vi "PH_Sequencer.ProcCases.vi"(0 "i ref in":refnum<vi>, 1 "selector":string, 2 "Data":T1, 3 "call cluster":T2={"Object"="", "Selector"="", "CallType"=enum."synchronous", "Async Object"="", "Async Selector"="", "Data Descriptor"="", "Data"=[], "Error #"=0, "Expire"=0}, 5 "error in (no error)":errorcluster) -> (14 "i ref out":refnum<vi>, 17 "answer cluster":T2={"Object"="", "Selector"="", "CallType"=enum."synchronous", "Async Object"="", "Async Selector"="", "Data Descriptor"="", "Data"=[], "Error #"=0, "Expire"=0}, 19 "error out":errorcluster)   [LabVIEW 2014, in "PH_Sequencer.lvlib"]
doc: "This method is called by a process from within the default case in the event loop. The methods of a class that are linked to events will be called from THIS method. Add your code here."
uses:
  PH_Sequencer.lvlib
  CSCore/CSSystem/CoreDefs/CoreDefs.call_type.ctl
  CSCore/BaseProcess/BaseProcess.descriptor string definition.ctl
  CSCore/CSSystem/CoreDefs/CoreDefs.rawDataType.ctl
  PH_Timing/PH_Timing.Slow Trigger Settings.ctl
  PH_Timing/PH_Timing.Phase FEs.ctl
  PH_Timing/PH_Timing.Timing Mode.ctl
  CSCore/CSSystem/CSSystemLib/CSSystemLib.object condition.ctl
  CSCore/CSSystem/CoreLib/CoreLib.string 2 byte array.vi
  CSCore/CSSystem/CoreLib/CoreLib.byte array 2 double.vi
  CSCore/CSSystem/CoreLib/CoreLib.byte array 2 short.vi
  CSCore/CSSystem/CoreLib/CoreLib.byte array 2 string.vi
  CSCore/BaseProcess/BaseProcess.lvlib
  CSCore/CAEObj/CAEObj.lvlib
  CSCore/CSSystem/CoreLib/CoreLib.lvlib
  CSCore/CSSystem/CSSystemLib/CSSystemLib.lvlib
  PH_Timing/PH_Timing.lvlib
  PH_Common/PH_Common.lvlib
  PH_PSDBController/PH_PSDBController.lvlib
  PH_PowerUnit_BaseClass/PH_PowerUnit_BaseClass.lvlib
  lib.lib/DimLVEvent/LVDimInterface/LVDimInterface.lvlib
  PH_StatusHandler/PH_StatusHandler.lvlib
  PH_PSDBWriter/PH_PSDBWriter.lvlib
  PH_SystemInformation/PH_SystemInformation.lvlib
  PH_BL-Master/PH_BL-Master.lvlib
  PH_4_Pos_Selector/PH_4_Pos_Selector.lvlib
  PH_BeamlineInformation/PH_BeamlineInformation.lvlib
  PH_BeamlineController/PH_BeamlineController.lvlib
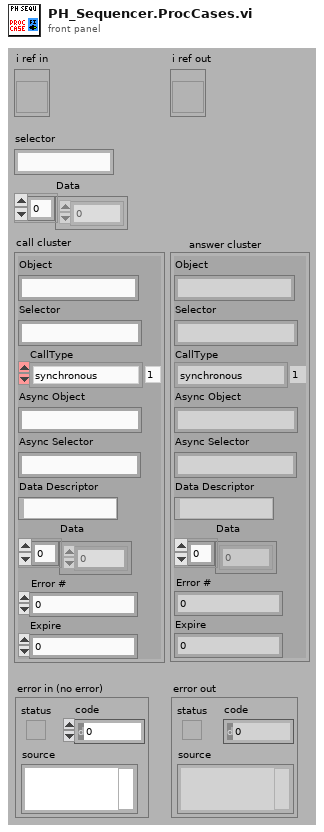
[diagram p1: front panel]
types:
  T1 = typedef "CoreDefs.rawDataType.ctl" = i8[]
  T2 = typedef "CoreDefs.call_type.ctl" = cluster{"Object":string, "Selector":string, "CallType":enum16{"simple", "synchronous", "asynchronous"}, "Async Object":string, "Async Selector":string, "Data Descriptor":T3, "Data":T1, "Error #":i32, "Expire":u32}
  T3 = typedef "BaseProcess.lvlib/BaseProcess.descriptor string definition.ctl" = string
  T4 = typedef "PH_Timing.lvlib/PH_Timing.Slow Trigger Settings.ctl" = cluster{"Delay":dbl, "externally triggered?":bool}
  T5 = typedef "PH_Timing.lvlib/PH_Timing.Phase FEs.ctl" = cluster{"Phase":dbl}
  T6 = typedef "PH_Timing.lvlib/PH_Timing.Timing Mode.ctl" = cluster{"T2":i16, "Modeselector":enum32{"10 Hz", "0.5 Hz", "Shot"}}
  T7 = typedef "PH_Sequencer.lvlib/PH_Sequencer.i attribute.ctl" = cluster{"GUI Refs":cluster{"Main Off":refnum<vi>, "Fire":refnum<vi>, "Status":refnum<vi>, "Ready":refnum<vi>, "Waiting Time":refnum<vi>, "Timeout":refnum<vi>, "PPMA Ready":refnum<vi>, "Sequencer SM State":refnum<vi>, "PPPA Ready":refnum<vi>, "Calorimeter":refnum<vi>, "Beamline Ready":refnum<vi>, "Clear Beamline":refnum<vi>, "Linkage PPMA Rods":refnum<vi>, "Linkage Current PA":refnum<vi>, "Linkage Current MA":refnum<vi>, "Timing Ready":refnum<vi>, "State Timing":refnum<vi>, "Force Timing":refnum<vi>, "PSDB Shot Comment":refnum<vi>, "State PA Backreflection":refnum<vi>, "Beamline Z6 Ready":refnum<vi>, "Clear Z6 Beamline":refnum<vi>, "Sequence length":refnum<vi>, "Timing Mode":refnum<vi>, "Slow Trigger Settings":refnum<vi>, "Experiment Description":refnum<vi>, "State PSDB":refnum<vi>, "PSDB Ready":refnum<vi>, "Set PSDB Settings":refnum<vi>, "Get PSDB Info":refnum<vi>, "Take Snapshot":refnum<vi>, "Shottype":refnum<vi>, "Experiment":refnum<vi>, "Phase Frontends":refnum<vi>, "PP 45mm PILC in use":refnum<vi>}, "Status Info":cluster{"Machine Status":T8, "WaitingTime":i32, "Timeout":bool}, "Readyness":cluster{"Ready to shot":bool, "PPMA Ready":bool, "PPPA Ready":bool, "BL Ready":bool, "Timing Ready":bool, "BL Z6 Ready":bool, "PSDBReady":bool}, "Instancenames":cluster{"PPMA Rods":string, "PP Current Meas":string, "PH Beamline Chief":string, "PA Backrefl Meas":string, "Z6 Beamline Chief":string}, "Data to read":bool, "Calorimeter":cluster{"Instancename":string, "On":bool, "linked":bool}, "Linkage":cluster{"PPMA Rods":bool, "PP Current Meas":bool, "PHELIX Beamline Chief":bool, "PA Backrefl Meas":bool, "Z6 Beamline Chief":bool}, "Timing":cluster{"Instance":string, "linked":bool, "Status":T8, "Timing Mode":T6, "Slow Trigger Settings":T4, "Info available":cluster{"ext SlowTrigger":bool, "T2":bool, "Mode":bool, "Delay Slow Trigger":bool, "Phase FEs":bool}, "FE Phase":T5}, "Service ID R2S":i32, "PSDB":cluster{"Controller Instance":string, "Controller Status":T8, "Controller linked":bool, "Settings acknowledged":bool, "Current Experiment ID":i16, "Current Shot Type":i16, "Current Comment":string, "Remember Settings":bool, "Write 2 early":bool}, "PSDB Data":cluster{"Main Off?":bool, "Sequence Length":dbl, "Sequence startet":timestamp}, "6P 4Q Positions":cluster{"Instancename":string, "linked":bool, "Position":T9}[], "PUs":T10[]}
  T8 = typedef "PH_StatusHandler.lvlib/PH_StatusHandler.Status.ctl" = i16
  T9 = typedef "PH_4_Pos_Selector.lvlib/PH_4_Pos_Selector.Position Selector.ctl" = u16
  T10 = typedef "PH_Sequencer.lvlib/PH_Sequencer.Head.ctl" = cluster{"PowerUnit":T11, "GUI Ref":refnum<vi>, "Information":T12, "linked?":bool, "GUI Ref Current Voltage":refnum<vi>}
  T11 = typedef "PH_PP_Common.lvlib/PH_PP_Common.PUs.ctl" = enum16{"no Info", "PA-19mm-1", "PA-19mm-2", "PA-45mm-PILC", "PA-45mm-MAIN", "MA-PU-1", "MA-PU-2", "MA-PU-3", "MA-PU-4", "MA-PU-5", "MA-PU-6", "MA-FR", "MA-PILC", "PA-45mm-DP"}
  T12 = typedef "PH_Sequencer.lvlib/PH_Sequencer.PU Information.ctl" = cluster{"State":T8, "Waiting Time [s]":dbl, "PU State SM":T13, "PU Timeout SM":T13}
  T13 = typedef "PH_PowerUnit_BaseClass.lvlib/PH_PowerUnit_BaseClass.SM States.ctl" = enum16{".", "Stand by", "Switch PU on", "Configure", "Set Default Voltage", "Set STANDBY", "Set READY", "Wait for Shot Cmd", "Open Dump Rods", "Open Ross Relais", "Close Ross Relais", "Switch PSU on", "Switch PSU off", "Charge", "Switch GD Channel on", "Close Dump Rods", "Rods-TO", "RR-TO", "PSU-TO", "Trigger-TO"}
  T14 = typedef "PH_SystemInformation.lvlib/PH_SystemInformation.i attribute.ctl" = cluster{"Laser Enabling":cluster{"GUI Ref":refnum<vi>, "Enabling State":T15}, "PreAmp Enabling":cluster{"GUI Ref":refnum<vi>, "Enabling State":T15}, "MainAmp Enabling":cluster{"GUI Ref":refnum<vi>, "Enabling State":T15}, "Emergency Off":cluster{"GUI Ref":refnum<vi>, "State":enum16{"no info", "off/false", "Alarm"}}, "Enabling Exp. 1":cluster{"GUI Ref":refnum<vi>, "Enabling State":T15}, "Enabling Exp. 2":cluster{"GUI Ref":refnum<vi>, "Enabling State":T15}, "Enabling Exp. 3":cluster{"GUI Ref":refnum<vi>, "Enabling State":T15}, "Enabling Exp. 4":cluster{"GUI Ref":refnum<vi>, "Enabling State":T15}, "Timing Mode":cluster{"GUI Ref":refnum<vi>, "PHELIX_Timing_Mode":enum32{"10 Hz", "0.5 Hz", "Shot"}}}
  T15 = typedef "PH_SystemInformation.lvlib/PH_SystemInformationEnabling State.ctl" = i32
  T16 = typedef "CSSystemLib.lvlib/CSSystemLib.object condition.ctl" = i32
  T17 = typedef "PH_PSDBWriter.lvlib/PH_PSDBWriter.PHELIX-Subsystems.ctl" = i32
  T18 = enum16{"Laser", "PreAmp", "MainAmp", "Exp 1", "Exp 2", "Exp 3", "Exp 4"}
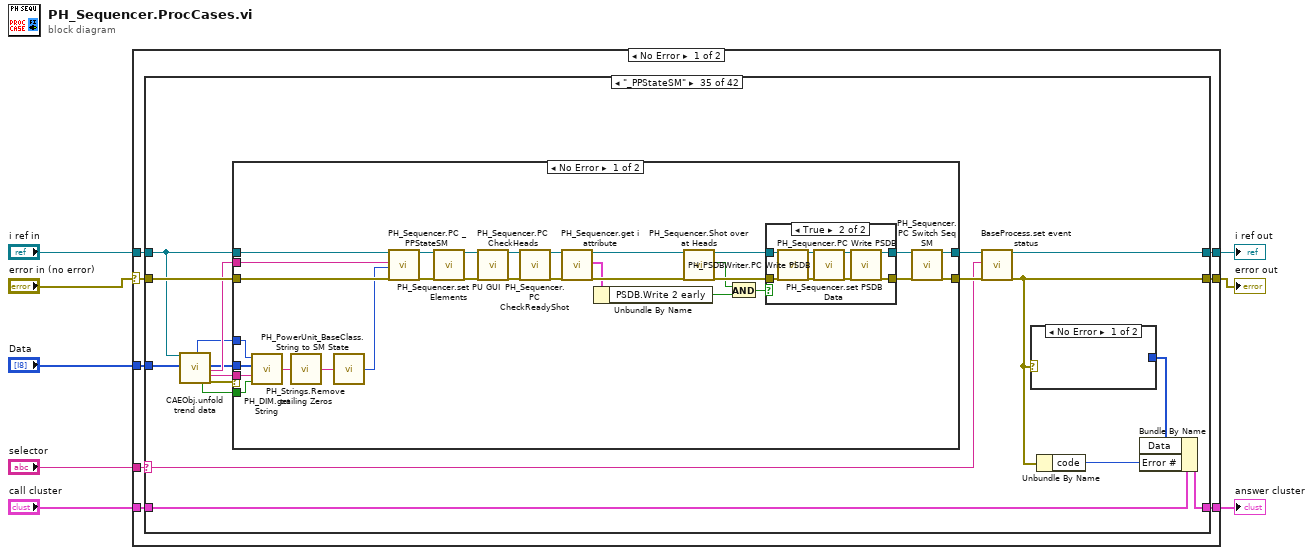
[diagram p0: block diagram]
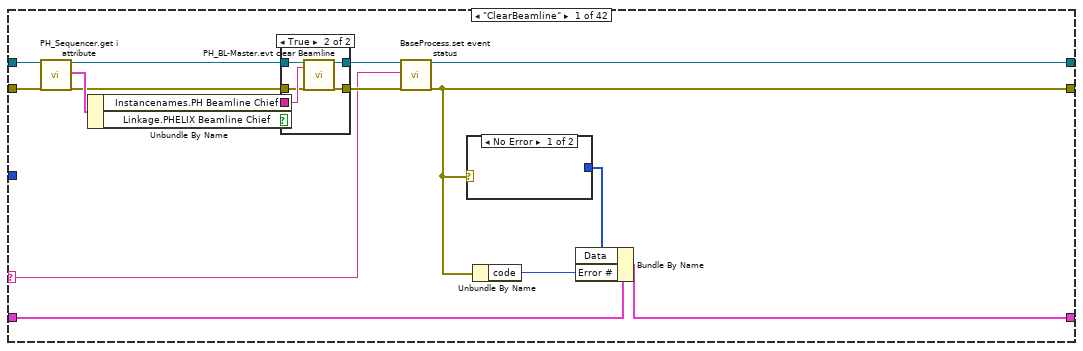
[diagram p2: hidden frame]
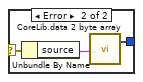
[diagram p4: hidden frame]
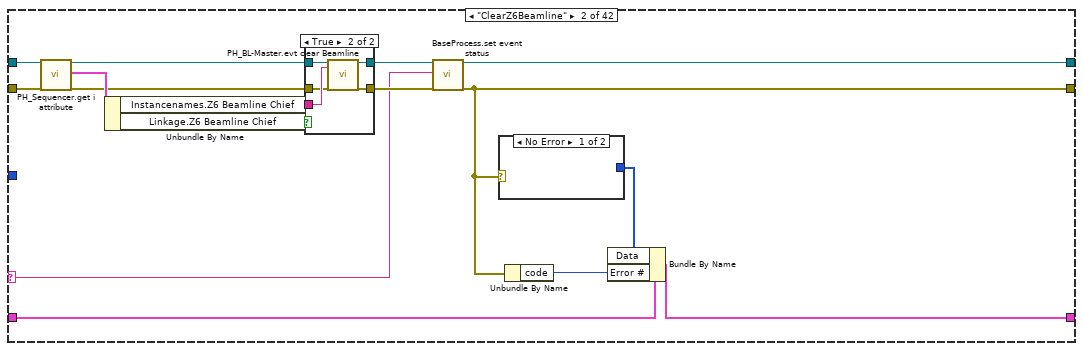
[diagram p5: hidden frame]
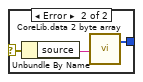
[diagram p7: hidden frame]
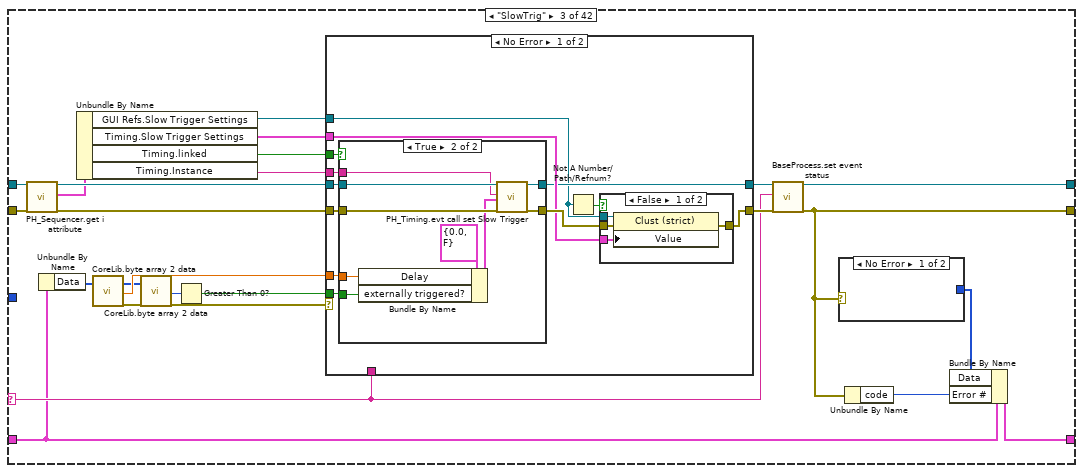
[diagram p8: hidden frame]
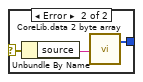
[diagram p9: hidden frame]
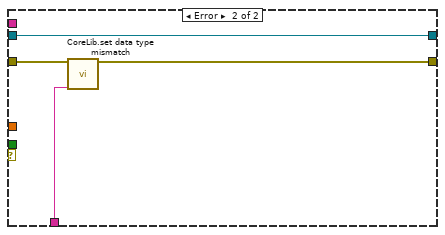
[diagram p12: hidden frame]
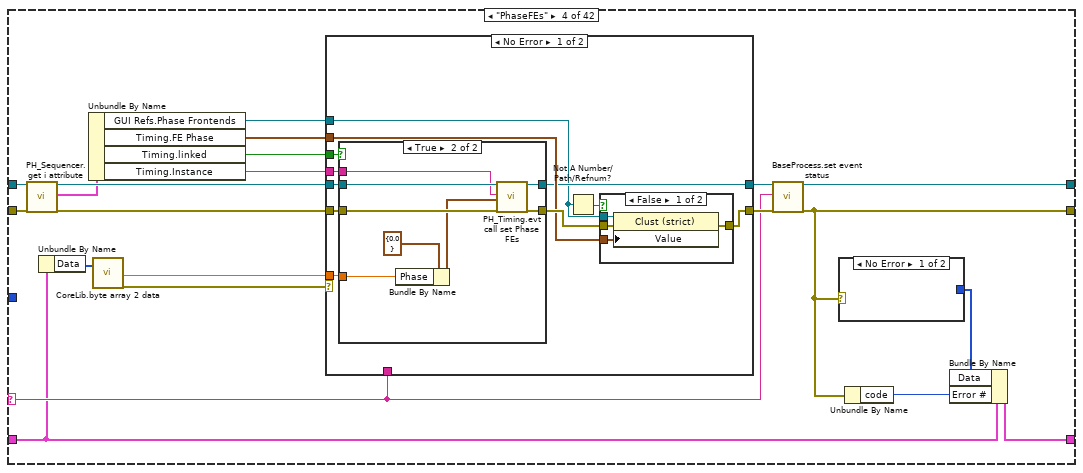
[diagram p13: hidden frame]
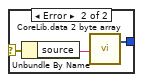
[diagram p14: hidden frame]
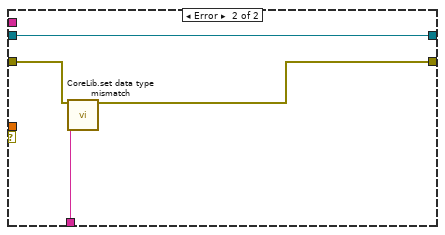
[diagram p17: hidden frame]
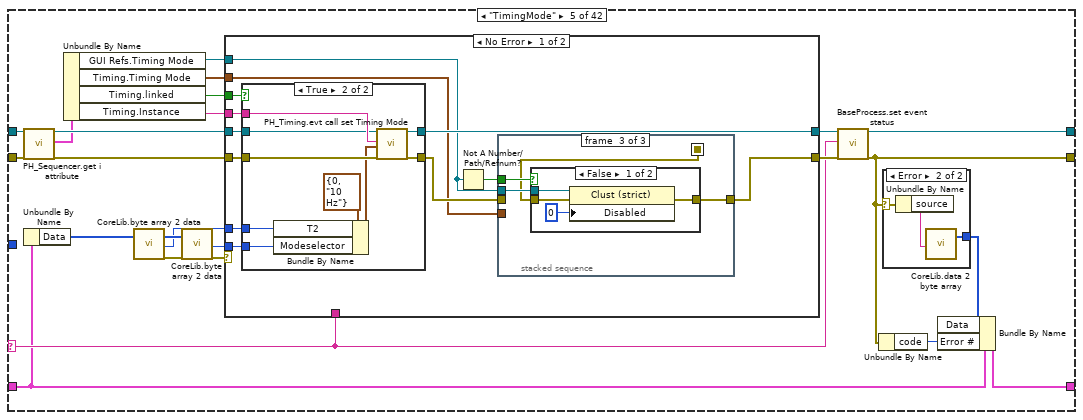
[diagram p18: hidden frame]
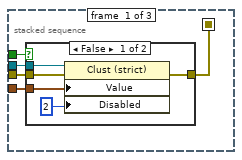
[diagram p20: hidden frame]
diagram:
  n1 = case shown="No Error" "error in (no error)" {
    selector: "error in (no error)" -> [w9 w1572]
    tunnel: "selector" -> [w16 _]
    tunnel: [w15 w1570] -> w7
    tunnel: "call cluster" -> [w14 w1570]
    tunnel: "i ref in" -> [w13 w1571]
    tunnel: [w12 w1571] -> w4
    tunnel: [w11 w1572] -> w3
    tunnel: "Data" -> [w10 _]
    frame No Error {
      n2 = case shown="\"_PPStateSM\"" w16 {
        selector: w16 -> [w18 w44 w87 w143 w200 w264 w298 w330 w363 w384 w404 w432 w449 w475 w513 w535 w549 w576 w605 w644 w675 w706 w754 w799 w854 w899 w952 w981 w1012 w1041 w1080 w1118 w1149 w1182 w1214 w1277 w1311 w1342 w1387 w1420 w1452 w1527]
        tunnel: w13 -> [w31 w57 w77 w137 w195 w272 w308 w338 w362 w376 w400 w431 w458 w484 w519 w543 w552 w581 w610 w648 w679 w710 w748 w791 w865 w910 w945 w974 w1004 w1055 w1077 w1115 w1146 w1179 w1210 w1273 w1307 w1355 w1380 w1413 w1448 w1513]
        tunnel: [w22 w48 w89 w145 w202 w266 w300 w332 w367 w388 w408 w436 w452 w477 w512 w537 w558 w587 w616 w641 w672 w703 w753 w798 w856 w901 w954 w983 w1009 w1042 w1083 w1121 w1152 w1185 w1216 w1279 w1313 w1344 w1389 w1422 w1454 w1530] -> w12
        tunnel: w14 -> [w20 w46 w85 w141 w198 w260 w297 w325 w364 w385 w405 w433 w445 w474 w505 w534 w550 w577 w606 w638 w669 w700 w750 w795 w852 w897 w950 w979 w1006 w1040 w1079 w1117 w1148 w1181 w1212 w1275 w1309 w1341 w1385 w1418 w1450 w1526]
        tunnel: [w19 w45 w86 w142 w199 w263 w296 w329 w365 w386 w406 w434 w450 w473 w510 w533 w556 w585 w614 w639 w670 w701 w751 w796 w853 w898 w951 w980 w1007 w1039 w1081 w1119 w1150 w1183 w1213 w1276 w1310 w1340 w1386 w1419 w1451 w1523] -> w15
        tunnel: w9 -> [w32 w58 w79 w139 w197 w271 w307 w337 w361 w378 w401 w430 w457 w486 w518 w542 w551 w579 w608 w647 w678 w709 w746 w790 w864 w909 w949 w978 w1015 w1056 w1088 w1126 w1157 w1190 w1221 w1284 w1318 w1357 w1384 w1417 w1447 w1512]
        tunnel: [w21 w47 w88 w144 w201 w265 w299 w331 w366 w387 w407 w435 w451 w476 w511 w536 w557 w586 w615 w640 w671 w702 w752 w797 w855 w900 w953 w982 w1008 w1043 w1082 w1120 w1151 w1184 w1215 w1278 w1312 w1343 w1388 w1421 w1453 w1529] -> w11
        tunnel: w10 -> [_ _ _ _ _ _ _ _ _ _ w399 _ _ _ _ _ _ _ _ w637 w668 w699 w749 w794 w866 w911 w946 w975 w1005 w1054 w1078 w1116 w1147 w1180 w1211 w1274 w1308 w1356 w1381 w1414 w1449 w1514]
        frame "ClearBeamline" {
          n3 = call "PH_Sequencer.get i attribute.vi"("i ref in"=w31, "error in (no error)"=w32) -> ("i ref out"=w29:refnum<vi>, "i attribute"=w30:T7, "error out"=w28:errorcluster)  [unwired: 15 in]
          n4 = Unbundle By Name(w30) -> ("Instancenames.PH Beamline Chief"=w27:string, "Linkage.PHELIX Beamline Chief"=w17:bool)
          n5 = case shown="True" w17 {
            tunnel: w29 -> [w34 w35]
            tunnel: w28 -> [w33 w36]
            tunnel: w27 -> [_ w37]
            tunnel: [w33 w38] -> w24
            tunnel: [w34 w39] -> w23
            frame False {
            }
            frame True {
              n6 = call "PH_BL-Master.evt clear Beamline.vi"("i ref in"=w35, "BL Instance"=w37, "error in (no error)"=w36) -> ("i ref out"=w39:refnum<vi>, "error out"=w38:errorcluster)  [unwired: 15 in]
            }
          }
          n7 = call "BaseProcess.set event status.vi"("i ref in"=w23, "EventStatus"=w18, "error in (no error)"=w24) -> ("i ref out"=w22:refnum<vi>, "error out"=w21:errorcluster)  [unwired: 14 in, 1 out]
          n8 = case shown="No Error" w21 {
            selector: w21 -> [_ w42]
            tunnel: [_ w40] -> w25
            frame No Error {
            }
            frame Error {
              n9 = Unbundle By Name(w42) -> ("source"=w41:string)
              n10 = call-poly "CoreLib.data 2 byte array.vi"("string"=w41) -> ("byteArray out"=w40:T1)  [unwired: 18 in]
            }
          }
          n11 = Unbundle By Name(w21) -> ("code"=w26:i32)
          n12 = Bundle By Name(cluster=w20, "Data"=w25, "Error #"=w26) -> (w19:T2)
        }
        frame "ClearZ6Beamline" {
          n13 = call "PH_Sequencer.get i attribute.vi"("i ref in"=w57, "error in (no error)"=w58) -> ("i ref out"=w55:refnum<vi>, "i attribute"=w56:T7, "error out"=w54:errorcluster)  [unwired: 15 in]
          n14 = Unbundle By Name(w56) -> ("Instancenames.Z6 Beamline Chief"=w53:string, "Linkage.Z6 Beamline Chief"=w43:bool)
          n15 = case shown="True" w43 {
            tunnel: w55 -> [w60 w61]
            tunnel: w54 -> [w59 w62]
            tunnel: w53 -> [_ w63]
            tunnel: [w59 w64] -> w50
            tunnel: [w60 w65] -> w49
            frame False {
            }
            frame True {
              n16 = call "PH_BL-Master.evt clear Beamline.vi"("i ref in"=w61, "BL Instance"=w63, "error in (no error)"=w62) -> ("i ref out"=w65:refnum<vi>, "error out"=w64:errorcluster)  [unwired: 15 in]
            }
          }
          n17 = call "BaseProcess.set event status.vi"("i ref in"=w49, "EventStatus"=w44, "error in (no error)"=w50) -> ("i ref out"=w48:refnum<vi>, "error out"=w47:errorcluster)  [unwired: 14 in, 1 out]
          n18 = case shown="No Error" w47 {
            selector: w47 -> [_ w68]
            tunnel: [_ w66] -> w51
            frame No Error {
            }
            frame Error {
              n19 = Unbundle By Name(w68) -> ("source"=w67:string)
              n20 = call-poly "CoreLib.data 2 byte array.vi"("string"=w67) -> ("byteArray out"=w66:T1)  [unwired: 18 in]
            }
          }
          n21 = Unbundle By Name(w47) -> ("code"=w52:i32)
          n22 = Bundle By Name(cluster=w46, "Data"=w51, "Error #"=w52) -> (w45:T2)
        }
        frame "SlowTrig" {
          n23 = call "PH_Sequencer.get i attribute.vi"("i ref in"=w77, "error in (no error)"=w79) -> ("i ref out"=w76:refnum<vi>, "i attribute"=w75:T7, "error out"=w78:errorcluster)  [unwired: 15 in]
          n24 = Unbundle By Name(w85) -> ("Data"=w72:T1)
          n25 = Unbundle By Name(w75) -> ("GUI Refs.Slow Trigger Settings"=w70:refnum<vi>, "Timing.Slow Trigger Settings"=w69:T4, "Timing.linked"=w73:bool, "Timing.Instance"=w74:string)
          n26 = call-poly "CoreLib.byte array 2 data.vi"("byteArray"=w72) -> ("byteArray out"=w82:T1, "d64"=w84:dbl, "error out"=w83:errorcluster)  [unwired: 16 in]
          n27 = call-poly "CoreLib.byte array 2 data.vi"("byteArray"=w82, "error in (no error)"=w83) -> ("i16"=w81:i16, "error out"=w71:errorcluster)  [unwired: 15 in, 1 out]
          n28 = Greater Than 0?(x=w81) -> (x > 0?=w80:bool)
          n29 = case shown="No Error" w71 {
            tunnel: [w99 w128] -> w90
            tunnel: w76 -> [w108 w128]
            tunnel: w78 -> [w107 w127]
            tunnel: [w101 w126] -> w91
            tunnel: w87 -> [_ w125]
            tunnel: w84 -> [w106 _]
            tunnel: w80 -> [w105 _]
            tunnel: w74 -> [w104 _]
            tunnel: w73 -> [w103 _]
            tunnel: w70 -> [w97 _]
            tunnel: w69 -> [w100 _]
            frame No Error {
              n30 = case shown="True" w103 {
                tunnel: w108 -> [w115 w124]
                tunnel: w107 -> [w114 w123]
                tunnel: w106 -> [_ w117]
                tunnel: [w114 w122] -> w102
                tunnel: [w115 w121] -> w99
                tunnel: w105 -> [_ w116]
                tunnel: w104 -> [_ w120]
                frame False {
                }
                frame True {
                  n31 = Bundle By Name(cluster=T4 {"Delay"=0.0, "externally triggered?"=FALSE} ("Slow Trigger Settings"), "Delay"=w117, "externally triggered?"=w116) -> (w119:T4)
                  n32 = call "PH_Timing.evt call set Slow Trigger.vi"("i ref in"=w124, "Instance"=w120, "Slow Trigger Settings"=w119, "error in (no error)"=w123) -> ("i ref out"=w121:refnum<vi>, "error out"=w122:errorcluster)  [unwired: 14 in]
                }
              }
              n33 = Not A Number/Path/Refnum?(number/path/refnum=w97) -> (NaN/Path/Refnum?=w98:bool)
              n34 = case shown="False" w98 {
                tunnel: w102 -> [w112 w113]
                tunnel: [w111 w113] -> w101
                tunnel: w97 -> [w110 _]
                tunnel: w100 -> [w109 _]
                frame False {
                  n35 = property class="Clust (strict)"(reference=w110, error in=w112, "Value"=w109) -> (error out=w111:errorcluster)  [unwired: 1 out]
                }
                frame True {
                }
              }
            }
            frame Error {
              n36 = call "CoreLib.set data type mismatch.vi"("error in (no error)"=w127, "error source"=w125) -> ("error out"=w126:errorcluster)  [unwired: 17 in]
            }
          }
          n37 = call "BaseProcess.set event status.vi"("i ref in"=w90, "EventStatus"=w87, "error in (no error)"=w91) -> ("i ref out"=w89:refnum<vi>, "error out"=w88:errorcluster)  [unwired: 14 in, 1 out]
          n38 = case shown="No Error" w88 {
            selector: w88 -> [_ w96]
            tunnel: [_ w94] -> w92
            frame No Error {
            }
            frame Error {
              n39 = Unbundle By Name(w96) -> ("source"=w95:string)
              n40 = call-poly "CoreLib.data 2 byte array.vi"("string"=w95) -> ("byteArray out"=w94:T1)  [unwired: 18 in]
            }
          }
          n41 = Unbundle By Name(w88) -> ("code"=w93:i32)
          n42 = Bundle By Name(cluster=w85, "Data"=w92, "Error #"=w93) -> (w86:T2)
        }
        frame "PhaseFEs" {
          n43 = call "PH_Sequencer.get i attribute.vi"("i ref in"=w137, "error in (no error)"=w139) -> ("i ref out"=w136:refnum<vi>, "i attribute"=w135:T7, "error out"=w138:errorcluster)  [unwired: 15 in]
          n44 = Unbundle By Name(w141) -> ("Data"=w132:T1)
          n45 = Unbundle By Name(w135) -> ("GUI Refs.Phase Frontends"=w131:refnum<vi>, "Timing.FE Phase"=w130:T5, "Timing.linked"=w133:bool, "Timing.Instance"=w134:string)
          n46 = call-poly "CoreLib.byte array 2 data.vi"("byteArray"=w132) -> ("d64"=w140:dbl, "error out"=w129:errorcluster)  [unwired: 16 in, 1 out]
          n47 = case shown="No Error" w129 {
            tunnel: [w155 w182] -> w146
            tunnel: w136 -> [w163 w182]
            tunnel: w138 -> [w162 w181]
            tunnel: [w157 w180] -> w147
            tunnel: w143 -> [_ w179]
            tunnel: w140 -> [w161 _]
            tunnel: w134 -> [w160 _]
            tunnel: w133 -> [w159 _]
            tunnel: w131 -> [w153 _]
            tunnel: w130 -> [w156 _]
            frame No Error {
              n48 = case shown="True" w159 {
                tunnel: w163 -> [w170 w178]
                tunnel: w162 -> [w169 w177]
                tunnel: w161 -> [_ w171]
                tunnel: [w169 w176] -> w158
                tunnel: [w170 w175] -> w155
                tunnel: w160 -> [_ w174]
                frame False {
                }
                frame True {
                  n49 = Bundle By Name(cluster=T5 {"Phase"=0.0} ("FE Phase"), "Phase"=w171) -> (w173:T5)
                  n50 = call "PH_Timing.evt call set Phase FEs.vi"("i ref in"=w178, "Instance"=w174, "Phase FEs"=w173, "error in (no error)"=w177) -> ("i ref out"=w175:refnum<vi>, "error out"=w176:errorcluster)  [unwired: 14 in]
                }
              }
              n51 = Not A Number/Path/Refnum?(number/path/refnum=w153) -> (NaN/Path/Refnum?=w154:bool)
              n52 = case shown="False" w154 {
                tunnel: w158 -> [w167 w168]
                tunnel: [w166 w168] -> w157
                tunnel: w153 -> [w165 _]
                tunnel: w156 -> [w164 _]
                frame False {
                  n53 = property class="Clust (strict)"(reference=w165, error in=w167, "Value"=w164) -> (error out=w166:errorcluster)  [unwired: 1 out]
                }
                frame True {
                }
              }
            }
            frame Error {
              n54 = call "CoreLib.set data type mismatch.vi"("error in (no error)"=w181, "error source"=w179) -> ("error out"=w180:errorcluster)  [unwired: 17 in]
            }
          }
          n55 = call "BaseProcess.set event status.vi"("i ref in"=w146, "EventStatus"=w143, "error in (no error)"=w147) -> ("i ref out"=w145:refnum<vi>, "error out"=w144:errorcluster)  [unwired: 14 in, 1 out]
          n56 = case shown="No Error" w144 {
            selector: w144 -> [_ w152]
            tunnel: [_ w150] -> w148
            frame No Error {
            }
            frame Error {
              n57 = Unbundle By Name(w152) -> ("source"=w151:string)
              n58 = call-poly "CoreLib.data 2 byte array.vi"("string"=w151) -> ("byteArray out"=w150:T1)  [unwired: 18 in]
            }
          }
          n59 = Unbundle By Name(w144) -> ("code"=w149:i32)
          n60 = Bundle By Name(cluster=w141, "Data"=w148, "Error #"=w149) -> (w142:T2)
        }
        frame "TimingMode" {
          n61 = call "PH_Sequencer.get i attribute.vi"("i ref in"=w195, "error in (no error)"=w197) -> ("i ref out"=w194:refnum<vi>, "i attribute"=w193:T7, "error out"=w196:errorcluster)  [unwired: 15 in]
          n62 = Unbundle By Name(w198) -> ("Data"=w184:T1)
          n63 = Unbundle By Name(w193) -> ("GUI Refs.Timing Mode"=w186:refnum<vi>, "Timing.Timing Mode"=w185:T6, "Timing.linked"=w191:bool, "Timing.Instance"=w192:string)
          n64 = call-poly "CoreLib.byte array 2 data.vi"("byteArray"=w184) -> ("byteArray out"=w189:T1, "i16"=w187:i16, "error out"=w190:errorcluster)  [unwired: 16 in]
          n65 = call-poly "CoreLib.byte array 2 data.vi"("byteArray"=w189, "error in (no error)"=w190) -> ("i16"=w183:i16, "error out"=w188:errorcluster)  [unwired: 15 in, 1 out]
          n66 = case shown="No Error" w188 {
            tunnel: [w219 w257] -> w203
            tunnel: w194 -> [w221 w257]
            tunnel: w196 -> [w220 w256]
            tunnel: [w210 w255] -> w204
            tunnel: w200 -> [_ w254]
            tunnel: w192 -> [w218 _]
            tunnel: w191 -> [w217 _]
            tunnel: w183 -> [w216 _]
            tunnel: w187 -> [w215 _]
            tunnel: w186 -> [w212 _]
            tunnel: w185 -> [w211 _]
            frame No Error {
              n67 = case shown="True" w217 {
                tunnel: w221 -> [w244 w249]
                tunnel: w220 -> [w243 w250]
                tunnel: [w243 w253] -> w213
                tunnel: [w244 w252] -> w219
                tunnel: w218 -> [_ w251]
                tunnel: w216 -> [_ w245]
                tunnel: w215 -> [_ w246]
                frame False {
                }
                frame True {
                  n68 = Bundle By Name(cluster=T6 {"T2"=0, "Modeselector"=enum."10 Hz"} ("Timing Mode"), "T2"=w246, "Modeselector"=w245) -> (w247:T6)
                  n69 = call "PH_Timing.evt call set Timing Mode.vi"("i ref in"=w249, "Instance"=w251, "Timing Mode"=w247, "error in (no error)"=w250) -> ("i ref out"=w252:refnum<vi>, "error out"=w253:errorcluster)  [unwired: 14 in]
                }
              }
              n70 = Not A Number/Path/Refnum?(number/path/refnum=w212) -> (NaN/Path/Refnum?=w214:bool)
              n71 = stacked-sequence {
                seq-local: [w222 _ _] -> [_ _ w235]
                tunnel: w214 -> [w226 _ w237]
                tunnel: w213 -> [w225 _ _]
                tunnel: w212 -> [w224 _ w236]
                tunnel: w211 -> [w223 _ _]
                tunnel: [_ _ w234] -> w210
                frame #0 {
                  n72 = case shown="False" w226 {
                    tunnel: w225 -> [w231 w232]
                    tunnel: [w230 w232] -> w222
                    tunnel: w224 -> [w229 _]
                    tunnel: w223 -> [w228 _]
                    frame False {
                      n73 = property class="Clust (strict)"(reference=w229, error in=w231, "Value"=w228, "Disabled"=u8 2) -> (error out=w230:errorcluster)  [unwired: 1 out]
                    }
                    frame True {
                    }
                  }
                }
                frame #1 {
                  n74 = Wait (ms)(milliseconds to wait=u32 1000) -> ()  [unwired: 1 out]
                }
                frame #2 {
                  n75 = case shown="False" w237 {
                    tunnel: w235 -> [w241 w242]
                    tunnel: [w240 w242] -> w234
                    tunnel: w236 -> [w239 _]
                    frame False {
                      n76 = property class="Clust (strict)"(reference=w239, error in=w241, "Disabled"=u8 0) -> (error out=w240:errorcluster)  [unwired: 1 out]
                    }
                    frame True {
                    }
                  }
                }
              }
            }
            frame Error {
              n77 = call "CoreLib.set data type mismatch.vi"("error in (no error)"=w256, "error source"=w254) -> ("error out"=w255:errorcluster)  [unwired: 17 in]
            }
          }
          n78 = call "BaseProcess.set event status.vi"("i ref in"=w203, "EventStatus"=w200, "error in (no error)"=w204) -> ("i ref out"=w202:refnum<vi>, "error out"=w201:errorcluster)  [unwired: 14 in, 1 out]
          n79 = Unbundle By Name(w201) -> ("code"=w206:i32)
          n80 = case shown="Error" w201 {
            selector: w201 -> [_ w209]
            tunnel: [_ w207] -> w205
            frame No Error {
            }
            frame Error {
              n81 = Unbundle By Name(w209) -> ("source"=w208:string)
              n82 = call-poly "CoreLib.data 2 byte array.vi"("string"=w208) -> ("byteArray out"=w207:T1)  [unwired: 18 in]
            }
          }
          n83 = Bundle By Name(cluster=w198, "Data"=w205, "Error #"=w206) -> (w199:T2)
        }
        frame "SetCalorimeter" {
          n84 = Unbundle By Name(w260) -> ("Data"=w262:T1)
          n85 = call-poly "CoreLib.byte array 2 data.vi"("byteArray"=w262) -> ("i16"=w261:i16, "error out"=w258:errorcluster)  [unwired: 16 in, 1 out]
          n86 = Greater Than 0?(x=w261) -> (x > 0?=w259:bool)
          n87 = case shown="No Error" w258 {
            tunnel: [w277 w284] -> w267
            tunnel: w272 -> [w279 w284]
            tunnel: w271 -> [w280 w283]
            tunnel: [w276 w282] -> w268
            tunnel: w264 -> [_ w281]
            tunnel: w259 -> [w278 _]
            frame No Error {
              n88 = call "PH_Sequencer.PC MA On.vi"("i ref in"=w279, "Calorimeter On"=w278, "error in (no error)"=w280) -> ("i ref out"=w277:refnum<vi>, "error out"=w276:errorcluster)  [unwired: 15 in]
            }
            frame Error {
              n89 = call "CoreLib.set data type mismatch.vi"("error in (no error)"=w283, "error source"=w281) -> ("error out"=w282:errorcluster)  [unwired: 17 in]
            }
          }
          n90 = call "BaseProcess.set event status.vi"("i ref in"=w267, "EventStatus"=w264, "error in (no error)"=w268) -> ("i ref out"=w266:refnum<vi>, "error out"=w265:errorcluster)  [unwired: 14 in, 1 out]
          n91 = case shown="No Error" w265 {
            selector: w265 -> [_ w275]
            tunnel: [_ w273] -> w269
            frame No Error {
            }
            frame Error {
              n92 = Unbundle By Name(w275) -> ("source"=w274:string)
              n93 = call-poly "CoreLib.data 2 byte array.vi"("string"=w274) -> ("byteArray out"=w273:T1)  [unwired: 18 in]
            }
          }
          n94 = Unbundle By Name(w265) -> ("code"=w270:i32)
          n95 = Bundle By Name(cluster=w260, "Data"=w269, "Error #"=w270) -> (w263:T2)
        }
        frame "MainOff" {
          n96 = call "PH_Sequencer.get i attribute.vi"("i ref in"=w308, "error in (no error)"=w307) -> ("i ref out"=w292:refnum<vi>, "i attribute"=w309:T7, "error out"=w293:errorcluster)  [unwired: 15 in]
          n97 = Unbundle By Name(w309) -> ("GUI Refs.Main Off"=w295:refnum<vi>)
          n98 = call "PH_GUI.set boolean GUI object.vi"("Boolean Knob GUI Ref"=w295, "Value"=FALSE, "error in (no error)"=w293) -> ("error out"=w291:errorcluster)  [unwired: 16 in]
          n99 = call "PH_Sequencer.get data to modify.vi"("i ref in"=w292, "error in (no error)"=w291) -> ("i ref out"=w286:refnum<vi>, "i attribute"=w288:T7, "timed out"=w287:bool, "error out"=w290:errorcluster)  [unwired: 14 in]
          n100 = case shown="False" w287 {
            tunnel: w290 -> [w316 w317]
            tunnel: [w315 w317] -> w289
            tunnel: w288 -> [w314 _]
            tunnel: w286 -> [w311 w318]
            tunnel: [w310 w318] -> w285
            frame False {
              n101 = Bundle By Name(cluster=w314, "PSDB Data.Main Off?"=TRUE) -> (w313:T7)
              n102 = call "PH_Sequencer.set modified data.vi"("i ref in"=w311, "i attribute"=w313, "error in (no error)"=w316) -> ("i ref out"=w310:refnum<vi>, "error out"=w315:errorcluster)  [unwired: 15 in]
            }
            frame True {
            }
          }
          n103 = call "PH_Sequencer.PC CheckReadyShot.vi"("i ref in"=w285, "error in (no error)"=w289) -> ("i ref out"=w306:refnum<vi>, "error out"=w305:errorcluster)  [unwired: 16 in]
          n104 = call "PH_Sequencer.set safe state.vi"("i ref in"=w306, "error in (no error)"=w305) -> ("i ref out"=w301:refnum<vi>, "error out"=w302:errorcluster)  [unwired: 16 in]
          n105 = call "BaseProcess.set event status.vi"("i ref in"=w301, "EventStatus"=w298, "error in (no error)"=w302) -> ("i ref out"=w300:refnum<vi>, "error out"=w299:errorcluster)  [unwired: 14 in, 1 out]
          n106 = Unbundle By Name(w299) -> ("code"=w304:i32)
          n107 = case shown="No Error" w299 {
            selector: w299 -> [_ w321]
            tunnel: [_ w319] -> w303
            frame No Error {
            }
            frame Error {
              n108 = Unbundle By Name(w321) -> ("source"=w320:string)
              n109 = call-poly "CoreLib.data 2 byte array.vi"("string"=w320) -> ("byteArray out"=w319:T1)  [unwired: 18 in]
            }
          }
          n110 = Bundle By Name(cluster=w297, "Data"=w303, "Error #"=w304) -> (w296:T2)
        }
        frame "PPTimeoutSM" {
          n111 = Unbundle By Name(w325) -> ("Data"=w328:T1)
          n112 = call-poly "CoreLib.byte array 2 data.vi"("byteArray"=w328) -> ("byteArray out"=w326:T1, "i16"=w323:i16, "error out"=w327:errorcluster)  [unwired: 16 in]
          n113 = call-poly "CoreLib.byte array 2 data.vi"("byteArray"=w326, "error in (no error)"=w327) -> ("i16"=w322:i16, "error out"=w324:errorcluster)  [unwired: 15 in, 1 out]
          n114 = case shown="No Error" w324 {
            tunnel: [w347 w355] -> w333
            tunnel: w338 -> [w351 w355]
            tunnel: w337 -> [w350 w354]
            tunnel: [w346 w353] -> w334
            tunnel: w330 -> [_ w352]
            tunnel: w323 -> [w349 _]
            tunnel: w322 -> [w348 _]
            frame No Error {
              n115 = call "PH_Sequencer.PC PPTimeoutSM.vi"("i ref in"=w351, "Power Unit"=w349, "SM Timeout"=w348, "error in (no error)"=w350) -> ("i ref out"=w345:refnum<vi>, "error out"=w343:errorcluster)  [unwired: 14 in]
              n116 = call "PH_Sequencer.set PU GUI Elements.vi"("VI in"=w345, "error in (no error)"=w343) -> ("VI out"=w344:refnum<vi>, "error out"=w342:errorcluster)  [unwired: 16 in]
              n117 = call "PH_Sequencer.PC CheckTOs.vi"("i ref in"=w344, "error in (no error)"=w342) -> ("i ref out"=w347:refnum<vi>, "error out"=w346:errorcluster)  [unwired: 16 in]
            }
            frame Error {
              n118 = call "CoreLib.set data type mismatch.vi"("error in (no error)"=w354, "error source"=w352) -> ("error out"=w353:errorcluster)  [unwired: 17 in]
            }
          }
          n119 = call "BaseProcess.set event status.vi"("i ref in"=w333, "EventStatus"=w330, "error in (no error)"=w334) -> ("i ref out"=w332:refnum<vi>, "error out"=w331:errorcluster)  [unwired: 14 in, 1 out]
          n120 = case shown="No Error" w331 {
            selector: w331 -> [_ w341]
            tunnel: [_ w339] -> w335
            frame No Error {
            }
            frame Error {
              n121 = Unbundle By Name(w341) -> ("source"=w340:string)
              n122 = call-poly "CoreLib.data 2 byte array.vi"("string"=w340) -> ("byteArray out"=w339:T1)  [unwired: 18 in]
            }
          }
          n123 = Unbundle By Name(w331) -> ("code"=w336:i32)
          n124 = Bundle By Name(cluster=w325, "Data"=w335, "Error #"=w336) -> (w329:T2)
        }
        frame "GetPSDBInfo" {
          n125 = call "PH_Sequencer.PC Get PSDB Info.vi"("i ref in"=w362, "error IO"=w361) -> ("i ref out"=w359:refnum<vi>, "error out"=w357:errorcluster)  [unwired: 16 in]
          n126 = call "PH_Sequencer.Acknowledge PSDB Settings.vi"("i ref in"=w359, "Settings acknowledged"=FALSE, "error IO"=w357) -> ("i ref out"=w358:refnum<vi>, "error out"=w356:errorcluster)  [unwired: 15 in]
          n127 = call "BaseProcess.set event status.vi"("i ref in"=w358, "EventStatus"=w363, "error in (no error)"=w356) -> ("i ref out"=w367:refnum<vi>, "error out"=w366:errorcluster)  [unwired: 14 in, 1 out]
          n128 = Unbundle By Name(w366) -> ("code"=w369:i32)
          n129 = case shown="Error" w366 {
            selector: w366 -> [_ w372]
            tunnel: [_ w370] -> w368
            frame No Error {
            }
            frame Error {
              n130 = Unbundle By Name(w372) -> ("source"=w371:string)
              n131 = call-poly "CoreLib.data 2 byte array.vi"("string"=w371) -> ("byteArray out"=w370:T1)  [unwired: 18 in]
            }
          }
          n132 = Bundle By Name(cluster=w364, "Data"=w368, "Error #"=w369) -> (w365:T2)
        }
        frame "GetPSDBSnapshot" {
          n133 = call "PH_Sequencer.get i attribute.vi"("i ref in"=w376, "error in (no error)"=w378) -> ("i ref out"=w375:refnum<vi>, "i attribute"=w374:T7, "error out"=w377:errorcluster)  [unwired: 15 in]
          n134 = Unbundle By Name(w374) -> ("PSDB.Controller Instance"=w373:string)
          n135 = call "PH_PSDBController.evt call take Snapshot.vi"("i ref in"=w375, "Instance"=w373, "error in (no error)"=w377) -> ("i ref out"=w382:refnum<vi>, "error out"=w380:errorcluster)  [unwired: 15 in]
          n136 = call "PH_Sequencer.Acknowledge PSDB Settings.vi"("i ref in"=w382, "Settings acknowledged"=FALSE, "error IO"=w380) -> ("i ref out"=w381:refnum<vi>, "error out"=w379:errorcluster)  [unwired: 15 in]
          n137 = call "BaseProcess.set event status.vi"("i ref in"=w381, "EventStatus"=w384, "error in (no error)"=w379) -> ("i ref out"=w388:refnum<vi>, "error out"=w387:errorcluster)  [unwired: 14 in, 1 out]
          n138 = Unbundle By Name(w387) -> ("code"=w390:i32)
          n139 = case shown="Error" w387 {
            selector: w387 -> [_ w393]
            tunnel: [_ w391] -> w389
            frame No Error {
            }
            frame Error {
              n140 = Unbundle By Name(w393) -> ("source"=w392:string)
              n141 = call-poly "CoreLib.data 2 byte array.vi"("string"=w392) -> ("byteArray out"=w391:T1)  [unwired: 18 in]
            }
          }
          n142 = Bundle By Name(cluster=w385, "Data"=w389, "Error #"=w390) -> (w386:T2)
        }
        frame "_PSDB-Info" {
          n143 = call "CAEObj.unfold trend data.vi"("i ref in"=w400, "raw trend data"=w399) -> ("no link"=w398:bool, "data"=w395:i8[], "serviceName"=w396:string, "typeDescriptor"=w394:string, "error out"=w397:errorcluster)  [unwired: 9 in, 4 out]
          n144 = case shown="No Error" w397 {
            tunnel: [w419 w423] -> w403
            tunnel: [w417 w422] -> w402
            tunnel: w401 -> [w416 w422]
            tunnel: w400 -> [w415 w423]
            tunnel: w396 -> [w413 _]
            tunnel: w395 -> [w414 _]
            tunnel: w398 -> [w412 _]
            tunnel: w394 -> [w411 _]
            frame No Error {
              n145 = call "PH_Sequencer.PC PSDB Info.vi"("i ref in"=w415, "data"=w414, "Service Name"=w413, "no link"=w412, "typeDescriptor"=w411, "error IO"=w416) -> ("i ref out"=w420:refnum<vi>, "error out"=w418:errorcluster)  [unwired: 12 in]
              n146 = call "PH_Sequencer.Acknowledge PSDB Settings.vi"("i ref in"=w420, "Settings acknowledged"=FALSE, "error IO"=w418) -> ("i ref out"=w419:refnum<vi>, "error out"=w417:errorcluster)  [unwired: 15 in]
            }
            frame Error {
            }
          }
          n147 = call "BaseProcess.set event status.vi"("i ref in"=w403, "EventStatus"=w404, "error in (no error)"=w402) -> ("i ref out"=w408:refnum<vi>, "error out"=w407:errorcluster)  [unwired: 14 in, 1 out]
          n148 = Unbundle By Name(w407) -> ("code"=w410:i32)
          n149 = case shown="Error" w407 {
            selector: w407 -> [_ w426]
            tunnel: [_ w424] -> w409
            frame No Error {
            }
            frame Error {
              n150 = Unbundle By Name(w426) -> ("source"=w425:string)
              n151 = call-poly "CoreLib.data 2 byte array.vi"("string"=w425) -> ("byteArray out"=w424:T1)  [unwired: 18 in]
            }
          }
          n152 = Bundle By Name(cluster=w405, "Data"=w409, "Error #"=w410) -> (w406:T2)
        }
        frame "SetPSDBSettings" {
          n153 = call "PH_Sequencer.Acknowledge PSDB Settings.vi"("i ref in"=w431, "Settings acknowledged"=TRUE, "error IO"=w430) -> ("i ref out"=w429:refnum<vi>, "error out"=w428:errorcluster)  [unwired: 15 in]
          n154 = call "BaseProcess.set event status.vi"("i ref in"=w429, "EventStatus"=w432, "error in (no error)"=w428) -> ("i ref out"=w436:refnum<vi>, "error out"=w435:errorcluster)  [unwired: 14 in, 1 out]
          n155 = Unbundle By Name(w435) -> ("code"=w438:i32)
          n156 = case shown="Error" w435 {
            selector: w435 -> [_ w441]
            tunnel: [_ w439] -> w437
            frame No Error {
            }
            frame Error {
              n157 = Unbundle By Name(w441) -> ("source"=w440:string)
              n158 = call-poly "CoreLib.data 2 byte array.vi"("string"=w440) -> ("byteArray out"=w439:T1)  [unwired: 18 in]
            }
          }
          n159 = Bundle By Name(cluster=w433, "Data"=w437, "Error #"=w438) -> (w434:T2)
        }
        frame "SetPPVoltage" {
          n160 = Unbundle By Name(w445) -> ("Data"=w448:T1)
          n161 = call-poly "CoreLib.byte array 2 data.vi"("byteArray"=w448) -> ("byteArray out"=w446:T1, "i16"=w444:i16, "error out"=w447:errorcluster)  [unwired: 16 in]
          n162 = call-poly "CoreLib.byte array 2 data.vi"("byteArray"=w446, "error in (no error)"=w447) -> ("d64"=w443:dbl, "error out"=w442:errorcluster)  [unwired: 15 in, 1 out]
          n163 = case shown="No Error" w442 {
            tunnel: [w464 w471] -> w453
            tunnel: w458 -> [w463 w471]
            tunnel: w457 -> [w462 w470]
            tunnel: [w465 w469] -> w454
            tunnel: w449 -> [_ w468]
            tunnel: w444 -> [w466 _]
            tunnel: w443 -> [w467 _]
            frame No Error {
              n164 = call "PH_PowerUnit_BaseClass.evt call Set Voltage.vi"("i ref in"=w463, "PowerUnit"=w466, "Voltage [V]"=w467, "error in (no error)"=w462) -> ("i ref out"=w464:refnum<vi>, "error out"=w465:errorcluster)  [unwired: 14 in]
            }
            frame Error {
              n165 = call "CoreLib.set data type mismatch.vi"("error in (no error)"=w470, "error source"=w468) -> ("error out"=w469:errorcluster)  [unwired: 17 in]
            }
          }
          n166 = call "BaseProcess.set event status.vi"("i ref in"=w453, "EventStatus"=w449, "error in (no error)"=w454) -> ("i ref out"=w452:refnum<vi>, "error out"=w451:errorcluster)  [unwired: 14 in, 1 out]
          n167 = case shown="No Error" w451 {
            selector: w451 -> [_ w461]
            tunnel: [_ w459] -> w455
            frame No Error {
            }
            frame Error {
              n168 = Unbundle By Name(w461) -> ("source"=w460:string)
              n169 = call-poly "CoreLib.data 2 byte array.vi"("string"=w460) -> ("byteArray out"=w459:T1)  [unwired: 18 in]
            }
          }
          n170 = Unbundle By Name(w451) -> ("code"=w456:i32)
          n171 = Bundle By Name(cluster=w445, "Data"=w455, "Error #"=w456) -> (w450:T2)
        }
        frame "Shot" {
          n172 = call "PH_Sequencer.get i attribute.vi"("i ref in"=w484, "error in (no error)"=w486) -> ("i ref out"=w483:refnum<vi>, "i attribute"=w482:T7, "error out"=w485:errorcluster)  [unwired: 15 in]
          n173 = Unbundle By Name(w482) -> ("Status Info.Timeout"=w472:bool)
          n174 = case shown="True" w472 {
            tunnel: [w493 w497] -> w488
            tunnel: [w492 w498] -> w487
            tunnel: w485 -> [w492 w501]
            tunnel: w483 -> [w493 w500]
            frame False {
            }
            frame True {
              n175 = call "PH_Sequencer.Reset TOs.vi"("i ref in"=w500, "error in (no error)"=w501) -> ("i ref out"=w495:refnum<vi>, "error out"=w499:errorcluster)  [unwired: 16 in]
              n176 = call "PH_Sequencer.set PU GUI Elements.vi"("VI in"=w495, "error in (no error)"=w499) -> ("VI out"=w494:refnum<vi>, "error out"=w496:errorcluster)  [unwired: 16 in]
              n177 = call "PH_Sequencer.PC CheckTOs.vi"("i ref in"=w494, "error in (no error)"=w496) -> ("i ref out"=w497:refnum<vi>, "error out"=w498:errorcluster)  [unwired: 16 in]
            }
          }
          n178 = call "PH_Sequencer.SCR Start Slow Devices.vi"("i ref in"=w488, "error in (no error)"=w487) -> ("i ref out"=w478:refnum<vi>, "error out"=w479:errorcluster)  [unwired: 16 in]
          n179 = call "BaseProcess.set event status.vi"("i ref in"=w478, "EventStatus"=w475, "error in (no error)"=w479) -> ("i ref out"=w477:refnum<vi>, "error out"=w476:errorcluster)  [unwired: 14 in, 1 out]
          n180 = case shown="No Error" w476 {
            selector: w476 -> [_ w491]
            tunnel: [_ w489] -> w480
            frame No Error {
            }
            frame Error {
              n181 = Unbundle By Name(w491) -> ("source"=w490:string)
              n182 = call-poly "CoreLib.data 2 byte array.vi"("string"=w490) -> ("byteArray out"=w489:T1)  [unwired: 18 in]
            }
          }
          n183 = Unbundle By Name(w476) -> ("code"=w481:i32)
          n184 = Bundle By Name(cluster=w474, "Data"=w480, "Error #"=w481) -> (w473:T2)
        }
        frame "SwitchPPon" {
          n185 = Unbundle By Name(w505) -> ("Data"=w509:T1)
          n186 = call-poly "CoreLib.byte array 2 data.vi"("byteArray"=w509) -> ("byteArray out"=w506:T1, "i16"=w504:i16, "error out"=w507:errorcluster)  [unwired: 16 in]
          n187 = call-poly "CoreLib.byte array 2 data.vi"("byteArray"=w506, "error in (no error)"=w507) -> ("i16"=w508:i16, "error out"=w502:errorcluster)  [unwired: 15 in, 1 out]
          n188 = Greater Than 0?(x=w508) -> (x > 0?=w503:bool)
          n189 = case shown="No Error" w502 {
            tunnel: [w527 w532] -> w514
            tunnel: w519 -> [w525 w532]
            tunnel: w518 -> [w524 w531]
            tunnel: [w528 w530] -> w515
            tunnel: w513 -> [_ w529]
            tunnel: w504 -> [w523 _]
            tunnel: w503 -> [w526 _]
            frame No Error {
              n190 = call "PH_PowerUnit_BaseClass.evt call PU on.vi"("i ref in"=w525, "PowerUnit"=w523, "PU on"=w526, "error in (no error)"=w524) -> ("i ref out"=w527:refnum<vi>, "error out"=w528:errorcluster)  [unwired: 14 in]
            }
            frame Error {
              n191 = call "CoreLib.set data type mismatch.vi"("error in (no error)"=w531, "error source"=w529) -> ("error out"=w530:errorcluster)  [unwired: 17 in]
            }
          }
          n192 = call "BaseProcess.set event status.vi"("i ref in"=w514, "EventStatus"=w513, "error in (no error)"=w515) -> ("i ref out"=w512:refnum<vi>, "error out"=w511:errorcluster)  [unwired: 14 in, 1 out]
          n193 = case shown="No Error" w511 {
            selector: w511 -> [_ w522]
            tunnel: [_ w520] -> w516
            frame No Error {
            }
            frame Error {
              n194 = Unbundle By Name(w522) -> ("source"=w521:string)
              n195 = call-poly "CoreLib.data 2 byte array.vi"("string"=w521) -> ("byteArray out"=w520:T1)  [unwired: 18 in]
            }
          }
          n196 = Unbundle By Name(w511) -> ("code"=w517:i32)
          n197 = Bundle By Name(cluster=w505, "Data"=w516, "Error #"=w517) -> (w510:T2)
        }
        frame "SwitchSeqSM" {
          n198 = call "PH_Sequencer.PC Switch Seq SM.vi"("i ref in"=w543, "error IO"=w542) -> ("i ref out"=w538:refnum<vi>, "error out"=w539:errorcluster)  [unwired: 16 in]
          n199 = call "BaseProcess.set event status.vi"("i ref in"=w538, "EventStatus"=w535, "error in (no error)"=w539) -> ("i ref out"=w537:refnum<vi>, "error out"=w536:errorcluster)  [unwired: 14 in, 1 out]
          n200 = case shown="No Error" w536 {
            selector: w536 -> [_ w546]
            tunnel: [_ w544] -> w540
            frame No Error {
            }
            frame Error {
              n201 = Unbundle By Name(w546) -> ("source"=w545:string)
              n202 = call-poly "CoreLib.data 2 byte array.vi"("string"=w545) -> ("byteArray out"=w544:T1)  [unwired: 18 in]
            }
          }
          n203 = Unbundle By Name(w536) -> ("code"=w541:i32)
          n204 = Bundle By Name(cluster=w534, "Data"=w540, "Error #"=w541) -> (w533:T2)
        }
        frame "SetShotComment" {
          n205 = Unbundle By Name(w550) -> ("Data"=w555:T1)
          n206 = call-poly "CoreLib.byte array 2 data.vi"("byteArray"=w555) -> ("string"=w553:string, "error out"=w554:errorcluster)  [unwired: 16 in, 1 out]
          n207 = case shown="No Error" w554 {
            tunnel: [w566 w572] -> w547
            tunnel: w552 -> [w562 w572]
            tunnel: w551 -> [w561 w571]
            tunnel: [w567 w570] -> w548
            tunnel: w549 -> [_ w569]
            tunnel: w553 -> [w563 _]
            frame No Error {
              n208 = call "PH_Sequencer.PC set Shot Comment.vi"("i ref in"=w562, "Shot Comment"=w563, "error IO"=w561) -> ("i ref out"=w565:refnum<vi>, "error out"=w564:errorcluster)  [unwired: 15 in]
              n209 = call "PH_Sequencer.Acknowledge PSDB Settings.vi"("i ref in"=w565, "Settings acknowledged"=FALSE, "error IO"=w564) -> ("i ref out"=w566:refnum<vi>, "error out"=w567:errorcluster)  [unwired: 15 in]
            }
            frame Error {
              n210 = call "CoreLib.set data type mismatch.vi"("error in (no error)"=w571, "error source"=w569) -> ("error out"=w570:errorcluster)  [unwired: 17 in]
            }
          }
          n211 = call "BaseProcess.set event status.vi"("i ref in"=w547, "EventStatus"=w549, "error in (no error)"=w548) -> ("i ref out"=w558:refnum<vi>, "error out"=w557:errorcluster)  [unwired: 14 in, 1 out]
          n212 = case shown="No Error" w557 {
            selector: w557 -> [_ w575]
            tunnel: [_ w573] -> w559
            frame No Error {
            }
            frame Error {
              n213 = Unbundle By Name(w575) -> ("source"=w574:string)
              n214 = call-poly "CoreLib.data 2 byte array.vi"("string"=w574) -> ("byteArray out"=w573:T1)  [unwired: 18 in]
            }
          }
          n215 = Unbundle By Name(w557) -> ("code"=w560:i32)
          n216 = Bundle By Name(cluster=w550, "Data"=w559, "Error #"=w560) -> (w556:T2)
        }
        frame "SetExpID" {
          n217 = Unbundle By Name(w577) -> ("Data"=w584:T1)
          n218 = call-poly "CoreLib.byte array 2 data.vi"("byteArray"=w584) -> ("i16"=w582:i16, "error out"=w583:errorcluster)  [unwired: 16 in, 1 out]
          n219 = case shown="No Error" w583 {
            tunnel: [w592 w601] -> w580
            tunnel: w581 -> [w596 w601]
            tunnel: w579 -> [w597 w600]
            tunnel: [w590 w599] -> w578
            tunnel: w576 -> [_ w598]
            tunnel: w582 -> [w595 _]
            frame No Error {
              n220 = call "PH_Sequencer.PC set Exp ID.vi"("i ref in"=w596, "Exp ID"=w595, "error IO"=w597) -> ("i ref out"=w593:refnum<vi>, "error out"=w591:errorcluster)  [unwired: 15 in]
              n221 = call "PH_Sequencer.Acknowledge PSDB Settings.vi"("i ref in"=w593, "Settings acknowledged"=FALSE, "error IO"=w591) -> ("i ref out"=w592:refnum<vi>, "error out"=w590:errorcluster)  [unwired: 15 in]
            }
            frame Error {
              n222 = call "CoreLib.set data type mismatch.vi"("error in (no error)"=w600, "error source"=w598) -> ("error out"=w599:errorcluster)  [unwired: 17 in]
            }
          }
          n223 = call "BaseProcess.set event status.vi"("i ref in"=w580, "EventStatus"=w576, "error in (no error)"=w578) -> ("i ref out"=w587:refnum<vi>, "error out"=w586:errorcluster)  [unwired: 14 in, 1 out]
          n224 = Unbundle By Name(w586) -> ("code"=w589:i32)
          n225 = case shown="Error" w586 {
            selector: w586 -> [_ w604]
            tunnel: [_ w602] -> w588
            frame No Error {
            }
            frame Error {
              n226 = Unbundle By Name(w604) -> ("source"=w603:string)
              n227 = call-poly "CoreLib.data 2 byte array.vi"("string"=w603) -> ("byteArray out"=w602:T1)  [unwired: 18 in]
            }
          }
          n228 = Bundle By Name(cluster=w577, "Data"=w588, "Error #"=w589) -> (w585:T2)
        }
        frame "SetShotType" {
          n229 = Unbundle By Name(w606) -> ("Data"=w613:T1)
          n230 = call-poly "CoreLib.byte array 2 data.vi"("byteArray"=w613) -> ("i16"=w611:i16, "error out"=w612:errorcluster)  [unwired: 16 in, 1 out]
          n231 = case shown="No Error" w612 {
            tunnel: [w621 w630] -> w609
            tunnel: w610 -> [w626 w630]
            tunnel: w608 -> [w625 w629]
            tunnel: [w619 w628] -> w607
            tunnel: w605 -> [_ w627]
            tunnel: w611 -> [w624 _]
            frame No Error {
              n232 = call "PH_Sequencer.PC set Shottypes.vi"("i ref in"=w626, "Shottype"=w624, "error IO"=w625) -> ("i ref out"=w622:refnum<vi>, "error out"=w620:errorcluster)  [unwired: 15 in]
              n233 = call "PH_Sequencer.Acknowledge PSDB Settings.vi"("i ref in"=w622, "Settings acknowledged"=FALSE, "error IO"=w620) -> ("i ref out"=w621:refnum<vi>, "error out"=w619:errorcluster)  [unwired: 15 in]
            }
            frame Error {
              n234 = call "CoreLib.set data type mismatch.vi"("error in (no error)"=w629, "error source"=w627) -> ("error out"=w628:errorcluster)  [unwired: 17 in]
            }
          }
          n235 = call "BaseProcess.set event status.vi"("i ref in"=w609, "EventStatus"=w605, "error in (no error)"=w607) -> ("i ref out"=w616:refnum<vi>, "error out"=w615:errorcluster)  [unwired: 14 in, 1 out]
          n236 = Unbundle By Name(w615) -> ("code"=w618:i32)
          n237 = case shown="Error" w615 {
            selector: w615 -> [_ w633]
            tunnel: [_ w631] -> w617
            frame No Error {
            }
            frame Error {
              n238 = Unbundle By Name(w633) -> ("source"=w632:string)
              n239 = call-poly "CoreLib.data 2 byte array.vi"("string"=w632) -> ("byteArray out"=w631:T1)  [unwired: 18 in]
            }
          }
          n240 = Bundle By Name(cluster=w606, "Data"=w617, "Error #"=w618) -> (w614:T2)
        }
        frame "_BeamlineState" {
          n241 = call "LVDimInterface.dim_unfold_data.vi"("rawData"=w637) -> ("data"=w634:i8[], "no link"=w635:bool, "error out"=w636:errorcluster)  [unwired: 15 in, 1 out]
          n242 = case shown="No Error" w636 {
            tunnel: [w661 w664] -> w642
            tunnel: w648 -> [w659 w664]
            tunnel: w647 -> [w660 w663]
            tunnel: [w662 w663] -> w643
            tunnel: w635 -> [w656 _]
            tunnel: w634 -> [w654 _]
            frame No Error {
              n243 = Not(x=w656) -> (.not. x?=w655:bool)
              n244 = Type Cast(type=0.0, x=w654) -> (*(type *) &x=w652:dbl)
              n245 = call "PH_Sequencer.set Beamline Settings.vi"("i ref in"=w659, "Beamline State"=w652, "linked?"=w655, "error in (no error)"=w660) -> ("i ref out"=w657:refnum<vi>, "error out"=w658:errorcluster)  [unwired: 14 in]
              n246 = call "PH_Sequencer.PC CheckReadyShot.vi"("i ref in"=w657, "error in (no error)"=w658) -> ("i ref out"=w661:refnum<vi>, "error out"=w662:errorcluster)  [unwired: 16 in]
            }
            frame Error {
            }
          }
          n247 = call "BaseProcess.set event status.vi"("i ref in"=w642, "EventStatus"=w644, "error in (no error)"=w643) -> ("i ref out"=w641:refnum<vi>, "error out"=w640:errorcluster)  [unwired: 14 in, 1 out]
          n248 = case shown="No Error" w640 {
            selector: w640 -> [_ w651]
            tunnel: [_ w649] -> w645
            frame No Error {
            }
            frame Error {
              n249 = Unbundle By Name(w651) -> ("source"=w650:string)
              n250 = call-poly "CoreLib.data 2 byte array.vi"("string"=w650) -> ("byteArray out"=w649:T1)  [unwired: 18 in]
            }
          }
          n251 = Unbundle By Name(w640) -> ("code"=w646:i32)
          n252 = Bundle By Name(cluster=w638, "Data"=w645, "Error #"=w646) -> (w639:T2)
        }
        frame "_Z6BeamlineState" {
          n253 = call "LVDimInterface.dim_unfold_data.vi"("rawData"=w668) -> ("data"=w665:i8[], "no link"=w666:bool, "error out"=w667:errorcluster)  [unwired: 15 in, 1 out]
          n254 = case shown="No Error" w667 {
            tunnel: [w692 w695] -> w673
            tunnel: w679 -> [w690 w695]
            tunnel: w678 -> [w691 w694]
            tunnel: [w693 w694] -> w674
            tunnel: w666 -> [w687 _]
            tunnel: w665 -> [w685 _]
            frame No Error {
              n255 = Not(x=w687) -> (.not. x?=w686:bool)
              n256 = Type Cast(type=0.0, x=w685) -> (*(type *) &x=w683:dbl)
              n257 = call "PH_Sequencer.set Z6 Beamline Settings.vi"("i ref in"=w690, "Z6 Beamline State"=w683, "linked?"=w686, "error in (no error)"=w691) -> ("i ref out"=w688:refnum<vi>, "error out"=w689:errorcluster)  [unwired: 14 in]
              n258 = call "PH_Sequencer.PC CheckReadyShot.vi"("i ref in"=w688, "error in (no error)"=w689) -> ("i ref out"=w692:refnum<vi>, "error out"=w693:errorcluster)  [unwired: 16 in]
            }
            frame Error {
            }
          }
          n259 = call "BaseProcess.set event status.vi"("i ref in"=w673, "EventStatus"=w675, "error in (no error)"=w674) -> ("i ref out"=w672:refnum<vi>, "error out"=w671:errorcluster)  [unwired: 14 in, 1 out]
          n260 = case shown="No Error" w671 {
            selector: w671 -> [_ w682]
            tunnel: [_ w680] -> w676
            frame No Error {
            }
            frame Error {
              n261 = Unbundle By Name(w682) -> ("source"=w681:string)
              n262 = call-poly "CoreLib.data 2 byte array.vi"("string"=w681) -> ("byteArray out"=w680:T1)  [unwired: 18 in]
            }
          }
          n263 = Unbundle By Name(w671) -> ("code"=w677:i32)
          n264 = Bundle By Name(cluster=w669, "Data"=w676, "Error #"=w677) -> (w670:T2)
        }
        frame "_ext_SlowTrigger" {
          n265 = call "LVDimInterface.dim_unfold_data.vi"("rawData"=w699) -> ("data"=w696:i8[], "no link"=w697:bool, "error out"=w698:errorcluster)  [unwired: 15 in, 1 out]
          n266 = case shown="No Error" w698 {
            tunnel: [w717 w741] -> w704
            tunnel: w710 -> [w722 w741]
            tunnel: w709 -> [w723 w740]
            tunnel: [w719 w740] -> w705
            tunnel: w697 -> [w720 _]
            tunnel: w696 -> [w725 _]
            frame No Error {
              n267 = Type Cast(type=i16 0, x=w725) -> (*(type *) &x=w714:i16)
              n268 = call "PH_Sequencer.get data to modify.vi"("i ref in"=w722, "error in (no error)"=w723) -> ("i ref out"=w718:refnum<vi>, "i attribute"=w716:T7, "timed out"=w715:bool, "error out"=w721:errorcluster)  [unwired: 14 in]
              n269 = case shown="False" w715 {
                tunnel: w721 -> [w734 w738]
                tunnel: w720 -> [w729 _]
                tunnel: [w730 w738] -> w719
                tunnel: w718 -> [w737 w739]
                tunnel: [w732 w739] -> w717
                tunnel: w716 -> [w736 _]
                tunnel: w714 -> [w727 _]
                frame False {
                  n270 = Greater Than 0?(x=w727) -> (x > 0?=w726:bool)
                  n271 = Not(x=w729) -> (.not. x?=w728:bool)
                  n272 = Bundle By Name(cluster=w736, "Timing.Slow Trigger Settings.externally triggered?"=w726, "Timing.Info available.ext SlowTrigger"=w728) -> (w735:T7)
                  n273 = call "PH_Sequencer.set modified data.vi"("i ref in"=w737, "i attribute"=w735, "error in (no error)"=w734) -> ("i ref out"=w733:refnum<vi>, "error out"=w731:errorcluster)  [unwired: 15 in]
                  n274 = call "PH_Sequencer.set Timing GUIs.vi"("i ref in"=w733, "error in"=w731) -> ("i ref out"=w732:refnum<vi>, "error out"=w730:errorcluster)  [unwired: 16 in]
                }
                frame True {
                }
              }
            }
            frame Error {
            }
          }
          n275 = call "BaseProcess.set event status.vi"("i ref in"=w704, "EventStatus"=w706, "error in (no error)"=w705) -> ("i ref out"=w703:refnum<vi>, "error out"=w702:errorcluster)  [unwired: 14 in, 1 out]
          n276 = Unbundle By Name(w702) -> ("code"=w708:i32)
          n277 = case shown="Error" w702 {
            selector: w702 -> [_ w713]
            tunnel: [_ w711] -> w707
            frame No Error {
            }
            frame Error {
              n278 = Unbundle By Name(w713) -> ("source"=w712:string)
              n279 = call-poly "CoreLib.data 2 byte array.vi"("string"=w712) -> ("byteArray out"=w711:T1)  [unwired: 18 in]
            }
          }
          n280 = Bundle By Name(cluster=w700, "Data"=w707, "Error #"=w708) -> (w701:T2)
        }
        frame "_T2" {
          n281 = call "LVDimInterface.dim_unfold_data.vi"("rawData"=w749) -> ("data"=w744:i8[], "no link"=w742:bool, "error out"=w743:errorcluster)  [unwired: 15 in, 1 out]
          n282 = case shown="No Error" w743 {
            tunnel: [w760 w783] -> w747
            tunnel: w748 -> [w765 w783]
            tunnel: w746 -> [w766 w782]
            tunnel: [w762 w782] -> w745
            tunnel: w742 -> [w763 _]
            tunnel: w744 -> [w768 _]
            frame No Error {
              n283 = call "PH_Sequencer.get data to modify.vi"("i ref in"=w765, "error in (no error)"=w766) -> ("i ref out"=w761:refnum<vi>, "i attribute"=w759:T7, "timed out"=w758:bool, "error out"=w764:errorcluster)  [unwired: 14 in]
              n284 = Type Cast(type=i16 0, x=w768) -> (*(type *) &x=w757:i16)
              n285 = case shown="False" w758 {
                tunnel: w764 -> [w776 w780]
                tunnel: w763 -> [w771 _]
                tunnel: [w772 w780] -> w762
                tunnel: w761 -> [w779 w781]
                tunnel: [w774 w781] -> w760
                tunnel: w759 -> [w778 _]
                tunnel: w757 -> [w769 _]
                frame False {
                  n286 = Not(x=w771) -> (.not. x?=w770:bool)
                  n287 = Bundle By Name(cluster=w778, "Timing.Timing Mode.T2"=w769, "Timing.Info available.T2"=w770) -> (w777:T7)
                  n288 = call "PH_Sequencer.set modified data.vi"("i ref in"=w779, "i attribute"=w777, "error in (no error)"=w776) -> ("i ref out"=w775:refnum<vi>, "error out"=w773:errorcluster)  [unwired: 15 in]
                  n289 = call "PH_Sequencer.set Timing GUIs.vi"("i ref in"=w775, "error in"=w773) -> ("i ref out"=w774:refnum<vi>, "error out"=w772:errorcluster)  [unwired: 16 in]
                }
                frame True {
                }
              }
            }
            frame Error {
            }
          }
          n290 = call "BaseProcess.set event status.vi"("i ref in"=w747, "EventStatus"=w754, "error in (no error)"=w745) -> ("i ref out"=w753:refnum<vi>, "error out"=w752:errorcluster)  [unwired: 14 in, 1 out]
          n291 = case shown="No Error" w752 {
            selector: w752 -> [_ w786]
            tunnel: [_ w784] -> w755
            frame No Error {
            }
            frame Error {
              n292 = Unbundle By Name(w786) -> ("source"=w785:string)
              n293 = call-poly "CoreLib.data 2 byte array.vi"("string"=w785) -> ("byteArray out"=w784:T1)  [unwired: 18 in]
            }
          }
          n294 = Unbundle By Name(w752) -> ("code"=w756:i32)
          n295 = Bundle By Name(cluster=w750, "Data"=w755, "Error #"=w756) -> (w751:T2)
        }
        frame "_Mode" {
          n296 = call "LVDimInterface.dim_unfold_data.vi"("rawData"=w794) -> ("data"=w787:i8[], "no link"=w788:bool, "error out"=w789:errorcluster)  [unwired: 15 in, 1 out]
          n297 = case shown="No Error" w789 {
            tunnel: [w805 w848] -> w793
            tunnel: w791 -> [w810 w848]
            tunnel: w790 -> [w811 w847]
            tunnel: [w807 w847] -> w792
            tunnel: w788 -> [w808 _]
            tunnel: w787 -> [w813 _]
            frame No Error {
              n298 = Type Cast(type=i16 0, x=w813) -> (*(type *) &x=w802:i16)
              n299 = call "PH_Sequencer.get data to modify.vi"("i ref in"=w810, "error in (no error)"=w811) -> ("i ref out"=w806:refnum<vi>, "i attribute"=w804:T7, "timed out"=w803:bool, "error out"=w809:errorcluster)  [unwired: 14 in]
              n300 = case shown="False" w803 {
                tunnel: w809 -> [w831 w845]
                tunnel: w808 -> [w828 _]
                tunnel: [w819 w845] -> w807
                tunnel: w806 -> [w835 w846]
                tunnel: [w820 w846] -> w805
                tunnel: w804 -> [w834 _]
                tunnel: w802 -> [w823 _]
                frame False {
                  n301 = Not(x=w828) -> (.not. x?=w826:bool)
                  n302 = Equal?(x=i16 -1, y=w823) -> (x = y?=w827:bool)
                  n303 = To Unsigned Long Integer(number=w823) -> (unsigned 32bit integer=w814:u32)
                  n304 = Select(t=FALSE, s=w827, f=w826) -> (s? t:f=w825:bool)
                  n305 = Bundle By Name(cluster=w834, "Timing.Timing Mode.Modeselector"=w814, "Timing.Info available.Mode"=w825) -> (w833:T7)
                  n306 = call "PH_Sequencer.set modified data.vi"("i ref in"=w835, "i attribute"=w833, "error in (no error)"=w831) -> ("i ref out"=w830:refnum<vi>, "error out"=w829:errorcluster)  [unwired: 15 in]
                  n307 = call "PH_Sequencer.set Timing GUIs.vi"("i ref in"=w830, "error in"=w829) -> ("i ref out"=w822:refnum<vi>, "error out"=w821:errorcluster)  [unwired: 16 in]
                  n308 = call "PH_SystemInformation.get data to modify.vi"("i ref in"=w822, "error in (no error)"=w821) -> ("i ref out"=w816:refnum<vi>, "i attribute"=w817:T14, "timed out"=w815:bool, "error out"=w818:errorcluster)  [unwired: 14 in]
                  n309 = case shown="False" w815 {
                    tunnel: w818 -> [w836 w843]
                    tunnel: w817 -> [w839 _]
                    tunnel: [w842 w843] -> w819
                    tunnel: w816 -> [w841 w844]
                    tunnel: [w840 w844] -> w820
                    tunnel: w814 -> [w837 _]
                    frame False {
                      n310 = Bundle By Name(cluster=w839, "Timing Mode.PHELIX_Timing_Mode"=w837) -> (w838:T14)
                      n311 = call "PH_SystemInformation.set modified data.vi"("i ref in"=w841, "i attribute"=w838, "error in (no error)"=w836) -> ("i ref out"=w840:refnum<vi>, "error out"=w842:errorcluster)  [unwired: 15 in]
                    }
                    frame True {
                    }
                  }
                }
                frame True {
                }
              }
            }
            frame Error {
            }
          }
          n312 = call "BaseProcess.set event status.vi"("i ref in"=w793, "EventStatus"=w799, "error in (no error)"=w792) -> ("i ref out"=w798:refnum<vi>, "error out"=w797:errorcluster)  [unwired: 14 in, 1 out]
          n313 = case shown="Error" w797 {
            selector: w797 -> [_ w851]
            tunnel: [_ w849] -> w800
            frame No Error {
            }
            frame Error {
              n314 = Unbundle By Name(w851) -> ("source"=w850:string)
              n315 = call-poly "CoreLib.data 2 byte array.vi"("string"=w850) -> ("byteArray out"=w849:T1)  [unwired: 18 in]
            }
          }
          n316 = Unbundle By Name(w797) -> ("code"=w801:i32)
          n317 = Bundle By Name(cluster=w795, "Data"=w800, "Error #"=w801) -> (w796:T2)
        }
        frame "_Delay_SlowTrigger" {
          n318 = call "LVDimInterface.dim_unfold_data.vi"("rawData"=w866) -> ("data"=w863:i8[], "no link"=w862:bool, "error out"=w861:errorcluster)  [unwired: 15 in, 1 out]
          n319 = case shown="No Error" w861 {
            tunnel: [w873 w896] -> w858
            tunnel: w865 -> [w878 w896]
            tunnel: w864 -> [w879 w895]
            tunnel: [w875 w895] -> w857
            tunnel: w862 -> [w876 _]
            tunnel: w863 -> [w881 _]
            frame No Error {
              n320 = call "PH_Sequencer.get data to modify.vi"("i ref in"=w878, "error in (no error)"=w879) -> ("i ref out"=w874:refnum<vi>, "i attribute"=w872:T7, "timed out"=w871:bool, "error out"=w877:errorcluster)  [unwired: 14 in]
              n321 = Type Cast(type=0.0, x=w881) -> (*(type *) &x=w870:dbl)
              n322 = case shown="False" w871 {
                tunnel: w877 -> [w888 w893]
                tunnel: w876 -> [w883 _]
                tunnel: [w884 w893] -> w875
                tunnel: w874 -> [w892 w894]
                tunnel: [w886 w894] -> w873
                tunnel: w872 -> [w891 _]
                tunnel: w870 -> [w889 _]
                frame False {
                  n323 = Not(x=w883) -> (.not. x?=w882:bool)
                  n324 = Bundle By Name(cluster=w891, "Timing.Slow Trigger Settings.Delay"=w889, "Timing.Info available.Delay Slow Trigger"=w882) -> (w890:T7)
                  n325 = call "PH_Sequencer.set modified data.vi"("i ref in"=w892, "i attribute"=w890, "error in (no error)"=w888) -> ("i ref out"=w887:refnum<vi>, "error out"=w885:errorcluster)  [unwired: 15 in]
                  n326 = call "PH_Sequencer.set Timing GUIs.vi"("i ref in"=w887, "error in"=w885) -> ("i ref out"=w886:refnum<vi>, "error out"=w884:errorcluster)  [unwired: 16 in]
                }
                frame True {
                }
              }
            }
            frame Error {
            }
          }
          n327 = call "BaseProcess.set event status.vi"("i ref in"=w858, "EventStatus"=w854, "error in (no error)"=w857) -> ("i ref out"=w856:refnum<vi>, "error out"=w855:errorcluster)  [unwired: 14 in, 1 out]
          n328 = case shown="Error" w855 {
            selector: w855 -> [_ w869]
            tunnel: [_ w867] -> w859
            frame No Error {
            }
            frame Error {
              n329 = Unbundle By Name(w869) -> ("source"=w868:string)
              n330 = call-poly "CoreLib.data 2 byte array.vi"("string"=w868) -> ("byteArray out"=w867:T1)  [unwired: 18 in]
            }
          }
          n331 = Unbundle By Name(w855) -> ("code"=w860:i32)
          n332 = Bundle By Name(cluster=w852, "Data"=w859, "Error #"=w860) -> (w853:T2)
        }
        frame "_Phase_FEs" {
          n333 = call "LVDimInterface.dim_unfold_data.vi"("rawData"=w911) -> ("data"=w908:i8[], "no link"=w907:bool, "error out"=w906:errorcluster)  [unwired: 15 in, 1 out]
          n334 = case shown="No Error" w906 {
            tunnel: [w918 w941] -> w903
            tunnel: w910 -> [w923 w941]
            tunnel: w909 -> [w924 w940]
            tunnel: [w920 w940] -> w902
            tunnel: w907 -> [w921 _]
            tunnel: w908 -> [w926 _]
            frame No Error {
              n335 = call "PH_Sequencer.get data to modify.vi"("i ref in"=w923, "error in (no error)"=w924) -> ("i ref out"=w919:refnum<vi>, "i attribute"=w917:T7, "timed out"=w916:bool, "error out"=w922:errorcluster)  [unwired: 14 in]
              n336 = Type Cast(type=0.0, x=w926) -> (*(type *) &x=w915:dbl)
              n337 = case shown="False" w916 {
                tunnel: w922 -> [w933 w938]
                tunnel: w921 -> [w928 _]
                tunnel: [w929 w938] -> w920
                tunnel: w919 -> [w937 w939]
                tunnel: [w931 w939] -> w918
                tunnel: w917 -> [w936 _]
                tunnel: w915 -> [w934 _]
                frame False {
                  n338 = Not(x=w928) -> (.not. x?=w927:bool)
                  n339 = Bundle By Name(cluster=w936, "Timing.FE Phase.Phase"=w934, "Timing.Info available.Phase FEs"=w927) -> (w935:T7)
                  n340 = call "PH_Sequencer.set modified data.vi"("i ref in"=w937, "i attribute"=w935, "error in (no error)"=w933) -> ("i ref out"=w932:refnum<vi>, "error out"=w930:errorcluster)  [unwired: 15 in]
                  n341 = call "PH_Sequencer.set Timing GUIs.vi"("i ref in"=w932, "error in"=w930) -> ("i ref out"=w931:refnum<vi>, "error out"=w929:errorcluster)  [unwired: 16 in]
                }
                frame True {
                }
              }
            }
            frame Error {
            }
          }
          n342 = call "BaseProcess.set event status.vi"("i ref in"=w903, "EventStatus"=w899, "error in (no error)"=w902) -> ("i ref out"=w901:refnum<vi>, "error out"=w900:errorcluster)  [unwired: 14 in, 1 out]
          n343 = case shown="Error" w900 {
            selector: w900 -> [_ w914]
            tunnel: [_ w912] -> w904
            frame No Error {
            }
            frame Error {
              n344 = Unbundle By Name(w914) -> ("source"=w913:string)
              n345 = call-poly "CoreLib.data 2 byte array.vi"("string"=w913) -> ("byteArray out"=w912:T1)  [unwired: 18 in]
            }
          }
          n346 = Unbundle By Name(w900) -> ("code"=w905:i32)
          n347 = Bundle By Name(cluster=w897, "Data"=w904, "Error #"=w905) -> (w898:T2)
        }
        frame "_Calorimeter" {
          n348 = call "CAEObj.unfold trend data.vi"("i ref in"=w945, "raw trend data"=w946) -> ("no link"=w943:bool, "data"=w942:i8[], "error out"=w944:errorcluster)  [unwired: 9 in, 6 out]
          n349 = case shown="No Error" w944 {
            tunnel: w945 -> [w965 w967]
            tunnel: [w964 w967] -> w948
            tunnel: w949 -> [w963 w966]
            tunnel: [w962 w966] -> w947
            tunnel: w943 -> [w958 _]
            tunnel: w942 -> [w959 _]
            frame No Error {
              w960 = T16 0 items=["undefined", "executing constructor", "_new: error", "_new: o.k.", "executing destructor"] ("condition")
              n350 = Type Cast(type=w960, x=w959) -> (*(type *) &x=w961:T16)
              n351 = Select(t=w960, s=w958, f=w961) -> (s? t:f=w957:T16)
              n352 = call "PH_Sequencer.set Calorimeter Settings.vi"("i ref in"=w965, "linked?"=w957, "error in (no error)"=w963) -> ("i ref out"=w964:refnum<vi>, "error out"=w962:errorcluster)  [unwired: 15 in]
            }
            frame Error {
            }
          }
          n353 = call "BaseProcess.set event status.vi"("i ref in"=w948, "EventStatus"=w952, "error in (no error)"=w947) -> ("i ref out"=w954:refnum<vi>, "error out"=w953:errorcluster)  [unwired: 14 in, 1 out]
          n354 = case shown="No Error" w953 {
            selector: w953 -> [_ w970]
            tunnel: [_ w968] -> w955
            frame No Error {
            }
            frame Error {
              n355 = Unbundle By Name(w970) -> ("source"=w969:string)
              n356 = call-poly "CoreLib.data 2 byte array.vi"("string"=w969) -> ("byteArray out"=w968:T1)  [unwired: 18 in]
            }
          }
          n357 = Unbundle By Name(w953) -> ("code"=w956:i32)
          n358 = Bundle By Name(cluster=w950, "Data"=w955, "Error #"=w956) -> (w951:T2)
        }
        frame "_CurrentMeas" {
          n359 = call "CAEObj.unfold trend data.vi"("i ref in"=w974, "raw trend data"=w975) -> ("no link"=w972:bool, "data"=w971:i8[], "error out"=w973:errorcluster)  [unwired: 9 in, 6 out]
          n360 = case shown="No Error" w973 {
            tunnel: w974 -> [w993 w996]
            tunnel: [w987 w996] -> w977
            tunnel: w978 -> [w994 w995]
            tunnel: [w986 w995] -> w976
            tunnel: w972 -> [w989 _]
            tunnel: w971 -> [w990 _]
            frame No Error {
              w991 = T16 0 items=["undefined", "executing constructor", "_new: error", "_new: o.k.", "executing destructor"] ("condition")
              n361 = Type Cast(type=w991, x=w990) -> (*(type *) &x=w992:T16)
              n362 = Select(t=w991, s=w989, f=w992) -> (s? t:f=w988:T16)
              n363 = call "PH_Sequencer.set PP CurrentMeas Settings.vi"("i ref in"=w993, "linked?"=w988, "error in (no error)"=w994) -> ("i ref out"=w987:refnum<vi>, "error out"=w986:errorcluster)  [unwired: 15 in]
            }
            frame Error {
            }
          }
          n364 = call "BaseProcess.set event status.vi"("i ref in"=w977, "EventStatus"=w981, "error in (no error)"=w976) -> ("i ref out"=w983:refnum<vi>, "error out"=w982:errorcluster)  [unwired: 14 in, 1 out]
          n365 = case shown="No Error" w982 {
            selector: w982 -> [_ w999]
            tunnel: [_ w997] -> w984
            frame No Error {
            }
            frame Error {
              n366 = Unbundle By Name(w999) -> ("source"=w998:string)
              n367 = call-poly "CoreLib.data 2 byte array.vi"("string"=w998) -> ("byteArray out"=w997:T1)  [unwired: 18 in]
            }
          }
          n368 = Unbundle By Name(w982) -> ("code"=w985:i32)
          n369 = Bundle By Name(cluster=w979, "Data"=w984, "Error #"=w985) -> (w980:T2)
        }
        frame "_PPInternalTiming" {
          n370 = call "CAEObj.unfold trend data.vi"("i ref in"=w1004, "raw trend data"=w1005) -> ("no link"=w1002:bool, "data"=w1001:i8[], "serviceName"=w1000:string, "error out"=w1003:errorcluster)  [unwired: 9 in, 5 out]
          n371 = case shown="No Error" w1003 {
            tunnel: [w1025 w1038] -> w1011
            tunnel: w1004 -> [w1034 w1038]
            tunnel: w1015 -> [w1033 w1037]
            tunnel: [w1024 w1036] -> w1010
            tunnel: w1012 -> [_ w1035]
            tunnel: w1002 -> [w1020 _]
            tunnel: w1001 -> [w1031 _]
            tunnel: w1000 -> [w1030 _]
            frame No Error {
              w1029 = 0.0
              n372 = Type Cast(type=w1029, x=w1031) -> (*(type *) &x=w1032:dbl)
              n373 = Select(t=w1029, s=w1020, f=w1032) -> (s? t:f=w1019:dbl)
              n374 = call "PH_Sequencer.PC PPInternalTiming.vi"("i ref in"=w1034, "Servicename"=w1030, "Waiting Time [s]"=w1019, "not linked?"=w1020, "error in (no error)"=w1033) -> ("i ref out"=w1022:refnum<vi>, "error out"=w1026:errorcluster)  [unwired: 13 in]
              n375 = call "PH_Sequencer.set PU GUI Elements.vi"("VI in"=w1022, "error in (no error)"=w1026) -> ("VI out"=w1021:refnum<vi>, "error out"=w1023:errorcluster)  [unwired: 16 in]
              n376 = call "PH_Sequencer.PC CheckWaitingTime.vi"("i ref in"=w1021, "error in (no error)"=w1023) -> ("i ref out"=w1028:refnum<vi>, "error out"=w1027:errorcluster)  [unwired: 16 in]
              n377 = call "PH_Sequencer.PC CheckReadyShot.vi"("i ref in"=w1028, "error in (no error)"=w1027) -> ("i ref out"=w1025:refnum<vi>, "error out"=w1024:errorcluster)  [unwired: 16 in]
            }
            frame Error {
              n378 = call "CoreLib.set data type mismatch.vi"("error in (no error)"=w1037, "error source"=w1035) -> ("error out"=w1036:errorcluster)  [unwired: 17 in]
            }
          }
          n379 = call "BaseProcess.set event status.vi"("i ref in"=w1011, "EventStatus"=w1012, "error in (no error)"=w1010) -> ("i ref out"=w1009:refnum<vi>, "error out"=w1008:errorcluster)  [unwired: 14 in, 1 out]
          n380 = Unbundle By Name(w1008) -> ("code"=w1014:i32)
          n381 = case shown="No Error" w1008 {
            selector: w1008 -> [_ w1018]
            tunnel: [_ w1016] -> w1013
            frame No Error {
            }
            frame Error {
              n382 = Unbundle By Name(w1018) -> ("source"=w1017:string)
              n383 = call-poly "CoreLib.data 2 byte array.vi"("string"=w1017) -> ("byteArray out"=w1016:T1)  [unwired: 18 in]
            }
          }
          n384 = Bundle By Name(cluster=w1006, "Data"=w1013, "Error #"=w1014) -> (w1007:T2)
        }
        frame "_PPMeasVolt" {
          n385 = call "CAEObj.unfold trend data.vi"("i ref in"=w1055, "raw trend data"=w1054) -> ("quality"=w1050:i32, "no link"=w1049:bool, "data"=w1051:i8[], "serviceName"=w1048:string, "typeDescriptor"=w1052:string, "error out"=w1053:errorcluster)  [unwired: 9 in, 3 out]
          n386 = case shown="No Error" w1053 {
            tunnel: [w1067 w1071] -> w1044
            tunnel: w1055 -> [w1069 w1071]
            tunnel: w1056 -> [w1068 w1070]
            tunnel: [w1066 w1070] -> w1045
            tunnel: w1052 -> [w1065 _]
            tunnel: w1051 -> [w1064 _]
            tunnel: w1050 -> [w1063 _]
            tunnel: w1049 -> [w1060 _]
            tunnel: w1048 -> [w1061 _]
            frame No Error {
              n387 = call "PH_DIM.get Double.vi"("no link"=w1060, "typeDescriptor"=w1065, "data"=w1064, "quality"=w1063) -> ("Value"=w1062:dbl)
              n388 = call "PH_Sequencer.PC _PPMeasVolt.vi"("i ref in"=w1069, "Tagname"=w1061, "Tagvalue"=w1062, "no link"=w1060, "error in (no error)"=w1068) -> ("i ref out"=w1067:refnum<vi>, "error out"=w1066:errorcluster)  [unwired: 13 in]
            }
            frame Error {
            }
          }
          n389 = call "BaseProcess.set event status.vi"("i ref in"=w1044, "EventStatus"=w1041, "error in (no error)"=w1045) -> ("i ref out"=w1042:refnum<vi>, "error out"=w1043:errorcluster)  [unwired: 14 in, 1 out]
          n390 = case shown="No Error" w1043 {
            selector: w1043 -> [_ w1059]
            tunnel: [_ w1057] -> w1046
            frame No Error {
            }
            frame Error {
              n391 = Unbundle By Name(w1059) -> ("source"=w1058:string)
              n392 = call-poly "CoreLib.data 2 byte array.vi"("string"=w1058) -> ("byteArray out"=w1057:T1)  [unwired: 18 in]
            }
          }
          n393 = Unbundle By Name(w1043) -> ("code"=w1047:i32)
          n394 = Bundle By Name(cluster=w1040, "Data"=w1046, "Error #"=w1047) -> (w1039:T2)
        }
        frame "_PPStatePU" {
          n395 = call "CAEObj.unfold trend data.vi"("i ref in"=w1077, "raw trend data"=w1078) -> ("no link"=w1075:bool, "data"=w1074:i8[], "serviceName"=w1073:string, "typeDescriptor"=w1072:string, "error out"=w1076:errorcluster)  [unwired: 9 in, 4 out]
          n396 = case shown="No Error" w1076 {
            tunnel: [w1106 w1110] -> w1084
            tunnel: w1077 -> [w1108 w1110]
            tunnel: w1088 -> [w1107 w1109]
            tunnel: [w1105 w1109] -> w1085
            tunnel: w1075 -> [w1100 _]
            tunnel: w1074 -> [w1103 _]
            tunnel: w1073 -> [w1104 _]
            tunnel: w1072 -> [w1102 _]
            frame No Error {
              n397 = call "PH_StatusHandler.get Status DIM Service.vi"("no link"=w1100, "typeDescriptor"=w1102, "data"=w1103) -> ("Status"=w1101:T8)  [unwired: 1 in]
              n398 = call "PH_Sequencer.PC PPStatePU.vi"("i ref in"=w1108, "Service Name"=w1104, "State"=w1101, "not linked?"=w1100, "error in (no error)"=w1107) -> ("i ref out"=w1098:refnum<vi>, "error out"=w1099:errorcluster)  [unwired: 13 in]
              n399 = call "PH_Sequencer.set PU GUI Elements.vi"("VI in"=w1098, "error in (no error)"=w1099) -> ("VI out"=w1095:refnum<vi>, "error out"=w1093:errorcluster)  [unwired: 16 in]
              n400 = call "PH_Sequencer.PC SetPPMAGUIElements.vi"("i ref in"=w1095, "error in (no error)"=w1093) -> ("i ref out"=w1096:refnum<vi>, "error out"=w1097:errorcluster)  [unwired: 16 in]
              n401 = call "PH_Sequencer.PC SetPPPAGUIElements.vi"("i ref in"=w1096, "error in (no error)"=w1097) -> ("i ref out"=w1094:refnum<vi>, "error out"=w1092:errorcluster)  [unwired: 16 in]
              n402 = call "PH_Sequencer.PC CheckMachineStatus.vi"("i ref in"=w1094, "error in (no error)"=w1092) -> ("i ref out"=w1106:refnum<vi>, "error out"=w1105:errorcluster)  [unwired: 16 in]
            }
            frame Error {
            }
          }
          n403 = call "BaseProcess.set event status.vi"("i ref in"=w1084, "EventStatus"=w1080, "error in (no error)"=w1085) -> ("i ref out"=w1083:refnum<vi>, "error out"=w1082:errorcluster)  [unwired: 14 in, 1 out]
          n404 = case shown="No Error" w1082 {
            selector: w1082 -> [_ w1091]
            tunnel: [_ w1089] -> w1086
            frame No Error {
            }
            frame Error {
              n405 = Unbundle By Name(w1091) -> ("source"=w1090:string)
              n406 = call-poly "CoreLib.data 2 byte array.vi"("string"=w1090) -> ("byteArray out"=w1089:T1)  [unwired: 18 in]
            }
          }
          n407 = Unbundle By Name(w1082) -> ("code"=w1087:i32)
          n408 = Bundle By Name(cluster=w1079, "Data"=w1086, "Error #"=w1087) -> (w1081:T2)
        }
        frame "_StateTiming" {
          n409 = call "CAEObj.unfold trend data.vi"("i ref in"=w1115, "raw trend data"=w1116) -> ("no link"=w1113:bool, "data"=w1112:i8[], "typeDescriptor"=w1111:string, "error out"=w1114:errorcluster)  [unwired: 9 in, 5 out]
          n410 = case shown="No Error" w1114 {
            tunnel: [w1132 w1141] -> w1122
            tunnel: w1115 -> [w1139 w1141]
            tunnel: w1126 -> [w1138 w1140]
            tunnel: [w1130 w1140] -> w1123
            tunnel: w1113 -> [w1134 _]
            tunnel: w1112 -> [w1137 _]
            tunnel: w1111 -> [w1136 _]
            frame No Error {
              n411 = call "PH_StatusHandler.get Status DIM Service.vi"("no link"=w1134, "typeDescriptor"=w1136, "data"=w1137) -> ("Status"=w1135:T8)  [unwired: 1 in]
              n412 = call "PH_Sequencer.PC StateTiming.vi"("i ref in"=w1139, "State"=w1135, "not linked?"=w1134, "error in (no error)"=w1138) -> ("i ref out"=w1133:refnum<vi>, "error out"=w1131:errorcluster)  [unwired: 14 in]
              n413 = call "PH_Sequencer.PC CheckReadyShot.vi"("i ref in"=w1133, "error in (no error)"=w1131) -> ("i ref out"=w1132:refnum<vi>, "error out"=w1130:errorcluster)  [unwired: 16 in]
            }
            frame Error {
            }
          }
          n414 = call "BaseProcess.set event status.vi"("i ref in"=w1122, "EventStatus"=w1118, "error in (no error)"=w1123) -> ("i ref out"=w1121:refnum<vi>, "error out"=w1120:errorcluster)  [unwired: 14 in, 1 out]
          n415 = case shown="No Error" w1120 {
            selector: w1120 -> [_ w1129]
            tunnel: [_ w1127] -> w1124
            frame No Error {
            }
            frame Error {
              n416 = Unbundle By Name(w1129) -> ("source"=w1128:string)
              n417 = call-poly "CoreLib.data 2 byte array.vi"("string"=w1128) -> ("byteArray out"=w1127:T1)  [unwired: 18 in]
            }
          }
          n418 = Unbundle By Name(w1120) -> ("code"=w1125:i32)
          n419 = Bundle By Name(cluster=w1117, "Data"=w1124, "Error #"=w1125) -> (w1119:T2)
        }
        frame "_StatusPSDB" {
          n420 = call "CAEObj.unfold trend data.vi"("i ref in"=w1146, "raw trend data"=w1147) -> ("no link"=w1144:bool, "data"=w1143:i8[], "typeDescriptor"=w1142:string, "error out"=w1145:errorcluster)  [unwired: 9 in, 5 out]
          n421 = case shown="No Error" w1145 {
            tunnel: [w1166 w1174] -> w1153
            tunnel: w1146 -> [w1172 w1174]
            tunnel: w1157 -> [w1171 w1173]
            tunnel: [w1165 w1173] -> w1154
            tunnel: w1144 -> [w1167 _]
            tunnel: w1143 -> [w1170 _]
            tunnel: w1142 -> [w1169 _]
            frame No Error {
              n422 = call "PH_StatusHandler.get Status DIM Service.vi"("no link"=w1167, "typeDescriptor"=w1169, "data"=w1170) -> ("Status"=w1168:T8)  [unwired: 1 in]
              n423 = call "PH_Sequencer.PC StatePSDB.vi"("i ref in"=w1172, "PSDB State"=w1168, "not linked?"=w1167, "error in (no error)"=w1171) -> ("i ref out"=w1164:refnum<vi>, "error out"=w1162:errorcluster)  [unwired: 14 in]
              n424 = call "PH_Sequencer.PC CheckPSDBReady.vi"("i ref in"=w1164, "error in (no error)"=w1162) -> ("i ref out"=w1163:refnum<vi>, "error out"=w1161:errorcluster)  [unwired: 16 in]
              n425 = call "PH_Sequencer.PC CheckReadyShot.vi"("i ref in"=w1163, "error in (no error)"=w1161) -> ("i ref out"=w1166:refnum<vi>, "error out"=w1165:errorcluster)  [unwired: 16 in]
            }
            frame Error {
            }
          }
          n426 = call "BaseProcess.set event status.vi"("i ref in"=w1153, "EventStatus"=w1149, "error in (no error)"=w1154) -> ("i ref out"=w1152:refnum<vi>, "error out"=w1151:errorcluster)  [unwired: 14 in, 1 out]
          n427 = case shown="No Error" w1151 {
            selector: w1151 -> [_ w1160]
            tunnel: [_ w1158] -> w1155
            frame No Error {
            }
            frame Error {
              n428 = Unbundle By Name(w1160) -> ("source"=w1159:string)
              n429 = call-poly "CoreLib.data 2 byte array.vi"("string"=w1159) -> ("byteArray out"=w1158:T1)  [unwired: 18 in]
            }
          }
          n430 = Unbundle By Name(w1151) -> ("code"=w1156:i32)
          n431 = Bundle By Name(cluster=w1148, "Data"=w1155, "Error #"=w1156) -> (w1150:T2)
        }
        frame "_StatusPABackrefl" {
          n432 = call "CAEObj.unfold trend data.vi"("i ref in"=w1179, "raw trend data"=w1180) -> ("no link"=w1177:bool, "data"=w1176:i8[], "typeDescriptor"=w1175:string, "error out"=w1178:errorcluster)  [unwired: 9 in, 5 out]
          n433 = case shown="No Error" w1178 {
            tunnel: [w1195 w1203] -> w1186
            tunnel: w1179 -> [w1201 w1203]
            tunnel: w1190 -> [w1200 w1202]
            tunnel: [w1194 w1202] -> w1187
            tunnel: w1177 -> [w1196 _]
            tunnel: w1176 -> [w1199 _]
            tunnel: w1175 -> [w1198 _]
            frame No Error {
              n434 = call "PH_StatusHandler.get Status DIM Service.vi"("no link"=w1196, "typeDescriptor"=w1198, "data"=w1199) -> ("Status"=w1197:T8)  [unwired: 1 in]
              n435 = call "PH_Sequencer.PC State PA Backrefl.vi"("i ref in"=w1201, "State"=w1197, "not linked?"=w1196, "error in (no error)"=w1200) -> ("i ref out"=w1195:refnum<vi>, "error out"=w1194:errorcluster)  [unwired: 14 in]
            }
            frame Error {
            }
          }
          n436 = call "BaseProcess.set event status.vi"("i ref in"=w1186, "EventStatus"=w1182, "error in (no error)"=w1187) -> ("i ref out"=w1185:refnum<vi>, "error out"=w1184:errorcluster)  [unwired: 14 in, 1 out]
          n437 = case shown="No Error" w1184 {
            selector: w1184 -> [_ w1193]
            tunnel: [_ w1191] -> w1188
            frame No Error {
            }
            frame Error {
              n438 = Unbundle By Name(w1193) -> ("source"=w1192:string)
              n439 = call-poly "CoreLib.data 2 byte array.vi"("string"=w1192) -> ("byteArray out"=w1191:T1)  [unwired: 18 in]
            }
          }
          n440 = Unbundle By Name(w1184) -> ("code"=w1189:i32)
          n441 = Bundle By Name(cluster=w1181, "Data"=w1188, "Error #"=w1189) -> (w1183:T2)
        }
        frame "_PPStateSM" {
          n442 = call "CAEObj.unfold trend data.vi"("i ref in"=w1210, "raw trend data"=w1211) -> ("quality"=w1204:i32, "no link"=w1205:bool, "data"=w1207:i8[], "serviceName"=w1208:string, "typeDescriptor"=w1206:string, "error out"=w1209:errorcluster)  [unwired: 9 in, 3 out]
          n443 = case shown="No Error" w1209 {
            tunnel: [w1246 w1266] -> w1217
            tunnel: w1210 -> [w1249 w1266]
            tunnel: w1221 -> [w1248 w1265]
            tunnel: [w1245 w1265] -> w1218
            tunnel: w1208 -> [w1251 _]
            tunnel: w1207 -> [w1254 _]
            tunnel: w1206 -> [w1253 _]
            tunnel: w1205 -> [w1247 _]
            tunnel: w1204 -> [w1252 _]
            frame No Error {
              n444 = call "PH_DIM.get String.vi"("no link"=w1247, "typeDescriptor"=w1253, "data"=w1254, "quality"=w1252) -> ("Output String"=w1250:string)
              n445 = call "PH_Strings.Remove trailing Zeros.vi"("Input String"=w1250) -> ("Output String"=w1233:string)
              n446 = call "PH_PowerUnit_BaseClass.String to SM State.vi"("SM State String"=w1233) -> ("SM State"=w1234:T13)
              n447 = call "PH_Sequencer.PC _PPStateSM.vi"("VI in"=w1249, "Service Name"=w1251, "PP SM State"=w1234, "error in (no error)"=w1248) -> ("VI out"=w1231:refnum<vi>, "error out"=w1232:errorcluster)  [unwired: 14 in]
              n448 = call "PH_Sequencer.set PU GUI Elements.vi"("VI in"=w1231, "error in (no error)"=w1232) -> ("VI out"=w1230:refnum<vi>, "error out"=w1229:errorcluster)  [unwired: 16 in]
              n449 = call "PH_Sequencer.PC CheckHeads.vi"("i ref in"=w1230, "error in (no error)"=w1229) -> ("i ref out"=w1227:refnum<vi>, "error out"=w1228:errorcluster)  [unwired: 16 in]
              n450 = call "PH_Sequencer.PC CheckReadyShot.vi"("i ref in"=w1227, "error in (no error)"=w1228) -> ("i ref out"=w1225:refnum<vi>, "error out"=w1226:errorcluster)  [unwired: 16 in]
              n451 = call "PH_Sequencer.get i attribute.vi"("i ref in"=w1225, "error in (no error)"=w1226) -> ("i ref out"=w1241:refnum<vi>, "i attribute"=w1240:T7, "error out"=w1242:errorcluster)  [unwired: 15 in]
              n452 = Unbundle By Name(w1240) -> ("PSDB.Write 2 early"=w1239:bool)
              n453 = call "PH_Sequencer.Shot over at Heads.vi"("i ref in"=w1241, "error in (no error)"=w1242) -> ("i ref out"=w1243:refnum<vi>, "Shot of all PUs passed"=w1238:bool, "error out"=w1244:errorcluster)  [unwired: 15 in]
              n454 = And(x=w1238, y=w1239) -> (x .and. y?=w1237:bool)
              n455 = case shown="True" w1237 {
                tunnel: [w1256 w1261] -> w1235
                tunnel: [w1255 w1259] -> w1236
                tunnel: w1243 -> [w1255 w1258]
                tunnel: w1244 -> [w1256 w1257]
                frame False {
                }
                frame True {
                  n456 = call "PH_Sequencer.PC Write PSDB.vi"("i ref in"=w1258, "error IO"=w1257) -> ("i ref out"=w1264:refnum<vi>, "error out"=w1263:errorcluster)  [unwired: 16 in]
                  n457 = call "PH_PSDBWriter.PC Write PSDB.vi"("i ref in"=w1264, "error IO"=w1263) -> ("i ref out"=w1260:refnum<vi>, "error out"=w1262:errorcluster)  [unwired: 16 in]
                  n458 = call "PH_Sequencer.set PSDB Data.vi"("i ref in"=w1260, "error in"=w1262) -> ("i ref out"=w1259:refnum<vi>, "error out"=w1261:errorcluster)  [unwired: 16 in]
                }
              }
              n459 = call "PH_Sequencer.PC Switch Seq SM.vi"("i ref in"=w1236, "error IO"=w1235) -> ("i ref out"=w1246:refnum<vi>, "error out"=w1245:errorcluster)  [unwired: 16 in]
            }
            frame Error {
            }
          }
          n460 = call "BaseProcess.set event status.vi"("i ref in"=w1217, "EventStatus"=w1214, "error in (no error)"=w1218) -> ("i ref out"=w1216:refnum<vi>, "error out"=w1215:errorcluster)  [unwired: 14 in, 1 out]
          n461 = case shown="No Error" w1215 {
            selector: w1215 -> [_ w1224]
            tunnel: [_ w1222] -> w1219
            frame No Error {
            }
            frame Error {
              n462 = Unbundle By Name(w1224) -> ("source"=w1223:string)
              n463 = call-poly "CoreLib.data 2 byte array.vi"("string"=w1223) -> ("byteArray out"=w1222:T1)  [unwired: 18 in]
            }
          }
          n464 = Unbundle By Name(w1215) -> ("code"=w1220:i32)
          n465 = Bundle By Name(cluster=w1212, "Data"=w1219, "Error #"=w1220) -> (w1213:T2)
        }
        frame "_Head_in_use" {
          n466 = call "CAEObj.unfold trend data.vi"("i ref in"=w1273, "raw trend data"=w1274) -> ("quality"=w1267:i32, "no link"=w1268:bool, "data"=w1270:i8[], "serviceName"=w1271:string, "typeDescriptor"=w1269:string, "error out"=w1272:errorcluster)  [unwired: 9 in, 3 out]
          n467 = case shown="No Error" w1272 {
            tunnel: [w1292 w1301] -> w1280
            tunnel: w1273 -> [w1294 w1301]
            tunnel: w1284 -> [w1293 w1300]
            tunnel: [w1291 w1300] -> w1281
            tunnel: w1271 -> [w1296 _]
            tunnel: w1270 -> [w1299 _]
            tunnel: w1269 -> [w1298 _]
            tunnel: w1268 -> [w1290 _]
            tunnel: w1267 -> [w1297 _]
            frame No Error {
              n468 = call "PH_DIM.get Boolean.vi"("no link"=w1290, "typeDescriptor"=w1298, "data"=w1299, "quality"=w1297) -> ("Value"=w1295:i32)
              n469 = Equal?(x=w1295, y=2) -> (x = y?=w1289:bool)
              n470 = call "PH_Sequencer.PC _Head_in_Use.vi"("VI in"=w1294, "Service Name in Use"=w1296, "in Use?"=w1289, "no link?"=w1290, "error in (no error)"=w1293) -> ("VI out"=w1292:refnum<vi>, "error out"=w1291:errorcluster)  [unwired: 13 in]
            }
            frame Error {
            }
          }
          n471 = call "BaseProcess.set event status.vi"("i ref in"=w1280, "EventStatus"=w1277, "error in (no error)"=w1281) -> ("i ref out"=w1279:refnum<vi>, "error out"=w1278:errorcluster)  [unwired: 14 in, 1 out]
          n472 = case shown="No Error" w1278 {
            selector: w1278 -> [_ w1287]
            tunnel: [_ w1285] -> w1282
            frame No Error {
            }
            frame Error {
              n473 = Unbundle By Name(w1287) -> ("source"=w1286:string)
              n474 = call-poly "CoreLib.data 2 byte array.vi"("string"=w1286) -> ("byteArray out"=w1285:T1)  [unwired: 18 in]
            }
          }
          n475 = Unbundle By Name(w1278) -> ("code"=w1283:i32)
          n476 = Bundle By Name(cluster=w1275, "Data"=w1282, "Error #"=w1283) -> (w1276:T2)
        }
        frame "PP_PA_45mm_PILC_in_use" {
          n477 = call "CAEObj.unfold trend data.vi"("i ref in"=w1307, "raw trend data"=w1308) -> ("quality"=w1302:i32, "no link"=w1303:bool, "data"=w1305:i8[], "typeDescriptor"=w1304:string, "error out"=w1306:errorcluster)  [unwired: 9 in, 4 out]
          n478 = case shown="No Error" w1306 {
            tunnel: [w1331 w1339] -> w1314
            tunnel: w1307 -> [w1333 w1339]
            tunnel: w1318 -> [w1332 w1338]
            tunnel: [w1328 w1338] -> w1315
            tunnel: w1305 -> [w1337 _]
            tunnel: w1304 -> [w1336 _]
            tunnel: w1303 -> [w1323 _]
            tunnel: w1302 -> [w1335 _]
            frame No Error {
              n479 = call "PH_DIM.get Boolean.vi"("no link"=w1323, "typeDescriptor"=w1336, "data"=w1337, "quality"=w1335) -> ("Value"=w1334:i32)
              n480 = Not(x=w1323) -> (.not. x?=w1322:bool)
              n481 = call "PH_Sequencer.get i attribute.vi"("i ref in"=w1333, "error in (no error)"=w1332) -> ("i ref out"=w1331:refnum<vi>, "i attribute"=w1326:T7, "error out"=w1330:errorcluster)  [unwired: 15 in]
              n482 = Equal?(x=w1334, y=2) -> (x = y?=w1327:bool)
              n483 = Unbundle By Name(w1326) -> ("GUI Refs.PP 45mm PILC in use"=w1325:refnum<vi>)
              n484 = call "PH_GUI.set boolean GUI object.vi"("Visible (true)"=w1322, "Boolean Knob GUI Ref"=w1325, "Value"=w1327, "error in (no error)"=w1330, "Tip Strip"="Indicates whether the \nPP PA 45mm PILC is in use") -> ("error out"=w1328:errorcluster)  [unwired: 14 in]
            }
            frame Error {
            }
          }
          n485 = call "BaseProcess.set event status.vi"("i ref in"=w1314, "EventStatus"=w1311, "error in (no error)"=w1315) -> ("i ref out"=w1313:refnum<vi>, "error out"=w1312:errorcluster)  [unwired: 14 in, 1 out]
          n486 = case shown="No Error" w1312 {
            selector: w1312 -> [_ w1321]
            tunnel: [_ w1319] -> w1316
            frame No Error {
            }
            frame Error {
              n487 = Unbundle By Name(w1321) -> ("source"=w1320:string)
              n488 = call-poly "CoreLib.data 2 byte array.vi"("string"=w1320) -> ("byteArray out"=w1319:T1)  [unwired: 18 in]
            }
          }
          n489 = Unbundle By Name(w1312) -> ("code"=w1317:i32)
          n490 = Bundle By Name(cluster=w1309, "Data"=w1316, "Error #"=w1317) -> (w1310:T2)
        }
        frame "_Head_voltage" {
          n491 = call "CAEObj.unfold trend data.vi"("i ref in"=w1355, "raw trend data"=w1356) -> ("quality"=w1353:i32, "no link"=w1350:bool, "data"=w1352:i8[], "serviceName"=w1349:string, "typeDescriptor"=w1351:string, "error out"=w1354:errorcluster)  [unwired: 9 in, 3 out]
          n492 = case shown="No Error" w1354 {
            tunnel: [w1370 w1376] -> w1345
            tunnel: w1355 -> [w1364 w1376]
            tunnel: w1357 -> [w1362 w1375]
            tunnel: [w1369 w1375] -> w1346
            tunnel: w1353 -> [w1374 _]
            tunnel: w1352 -> [w1373 _]
            tunnel: w1351 -> [w1372 _]
            tunnel: w1350 -> [w1365 _]
            tunnel: w1349 -> [w1367 _]
            frame No Error {
              n493 = call "PH_DIM.get Double.vi"("no link"=w1365, "typeDescriptor"=w1372, "data"=w1373, "quality"=w1374) -> ("Value"=w1366:dbl)
              n494 = call "PH_BeamlineInformation.PC _Voltage of Head.vi"("i ref in"=w1364, "Voltage Service Name"=w1367, "Voltage [V]"=w1366, "no link?"=w1365, "error in (no error)"=w1362) -> ("i ref out"=w1363:refnum<vi>, "error out"=w1361:errorcluster)  [unwired: 13 in]
              n495 = call "PH_Sequencer.PC SetPPMAGUIElements.vi"("i ref in"=w1363, "error in (no error)"=w1361) -> ("i ref out"=w1368:refnum<vi>, "error out"=w1371:errorcluster)  [unwired: 16 in]
              n496 = call "PH_Sequencer.PC SetPPPAGUIElements.vi"("i ref in"=w1368, "error in (no error)"=w1371) -> ("i ref out"=w1370:refnum<vi>, "error out"=w1369:errorcluster)  [unwired: 16 in]
            }
            frame Error {
            }
          }
          n497 = call "BaseProcess.set event status.vi"("i ref in"=w1345, "EventStatus"=w1342, "error in (no error)"=w1346) -> ("i ref out"=w1344:refnum<vi>, "error out"=w1343:errorcluster)  [unwired: 14 in, 1 out]
          n498 = case shown="No Error" w1343 {
            selector: w1343 -> [_ w1360]
            tunnel: [_ w1358] -> w1347
            frame No Error {
            }
            frame Error {
              n499 = Unbundle By Name(w1360) -> ("source"=w1359:string)
              n500 = call-poly "CoreLib.data 2 byte array.vi"("string"=w1359) -> ("byteArray out"=w1358:T1)  [unwired: 18 in]
            }
          }
          n501 = Unbundle By Name(w1343) -> ("code"=w1348:i32)
          n502 = Bundle By Name(cluster=w1341, "Data"=w1347, "Error #"=w1348) -> (w1340:T2)
        }
        frame "_linkRods" {
          n503 = call "CAEObj.unfold trend data.vi"("i ref in"=w1380, "raw trend data"=w1381) -> ("no link"=w1378:bool, "data"=w1377:i8[], "error out"=w1379:errorcluster)  [unwired: 9 in, 6 out]
          n504 = case shown="No Error" w1379 {
            tunnel: w1380 -> [w1402 w1404]
            tunnel: [w1394 w1404] -> w1383
            tunnel: w1384 -> [w1401 w1403]
            tunnel: [w1392 w1403] -> w1382
            tunnel: w1378 -> [w1400 _]
            tunnel: w1377 -> [w1396 _]
            frame No Error {
              w1397 = T16 0 items=["undefined", "executing constructor", "_new: error", "_new: o.k.", "executing destructor"] ("condition")
              n505 = Type Cast(type=w1397, x=w1396) -> (*(type *) &x=w1399:T16)
              n506 = Select(t=w1397, s=w1400, f=w1399) -> (s? t:f=w1398:T16)
              n507 = call "PH_Sequencer.set PPMA Rods Settings.vi"("i ref in"=w1402, "condition"=w1398, "error in (no error)"=w1401) -> ("i ref out"=w1395:refnum<vi>, "error out"=w1393:errorcluster)  [unwired: 15 in]
              n508 = call "PH_Sequencer.PC SetPPMAGUIElements.vi"("i ref in"=w1395, "error in (no error)"=w1393) -> ("i ref out"=w1394:refnum<vi>, "error out"=w1392:errorcluster)  [unwired: 16 in]
            }
            frame Error {
            }
          }
          n509 = call "BaseProcess.set event status.vi"("i ref in"=w1383, "EventStatus"=w1387, "error in (no error)"=w1382) -> ("i ref out"=w1389:refnum<vi>, "error out"=w1388:errorcluster)  [unwired: 14 in, 1 out]
          n510 = Unbundle By Name(w1388) -> ("code"=w1391:i32)
          n511 = case shown="No Error" w1388 {
            selector: w1388 -> [_ w1407]
            tunnel: [_ w1405] -> w1390
            frame No Error {
            }
            frame Error {
              n512 = Unbundle By Name(w1407) -> ("source"=w1406:string)
              n513 = call-poly "CoreLib.data 2 byte array.vi"("string"=w1406) -> ("byteArray out"=w1405:T1)  [unwired: 18 in]
            }
          }
          n514 = Bundle By Name(cluster=w1385, "Data"=w1390, "Error #"=w1391) -> (w1386:T2)
        }
        frame "_6P_4Q_Position" {
          n515 = call "CAEObj.unfold trend data.vi"("i ref in"=w1413, "raw trend data"=w1414) -> ("no link"=w1411:bool, "data"=w1410:i8[], "serviceName"=w1409:string, "typeDescriptor"=w1408:string, "error out"=w1412:errorcluster)  [unwired: 9 in, 4 out]
          n516 = case shown="No Error" w1412 {
            tunnel: w1413 -> [w1434 w1436]
            tunnel: [w1431 w1436] -> w1416
            tunnel: w1417 -> [w1433 w1435]
            tunnel: [w1432 w1435] -> w1415
            tunnel: w1411 -> [w1428 _]
            tunnel: w1410 -> [w1427 _]
            tunnel: w1409 -> [w1430 _]
            tunnel: w1408 -> [w1426 _]
            frame No Error {
              n517 = call "PH_4_Pos_Selector.get 6P 4Q Position DIM Service.vi"("no link"=w1428, "typeDescriptor"=w1426, "data"=w1427) -> ("Position"=w1425:T9)  [unwired: 1 in]
              n518 = Not(x=w1428) -> (.not. x?=w1429:bool)
              n519 = call "PH_Sequencer.PC _6P_4Q_Pos.vi"("VI in"=w1434, "Selector"=w1425, "serviceName"=w1430, "linked?"=w1429, "error in"=w1433) -> ("VI out"=w1431:refnum<vi>, "error out"=w1432:errorcluster)  [unwired: 13 in]
            }
            frame Error {
            }
          }
          n520 = call "BaseProcess.set event status.vi"("i ref in"=w1416, "EventStatus"=w1420, "error in (no error)"=w1415) -> ("i ref out"=w1422:refnum<vi>, "error out"=w1421:errorcluster)  [unwired: 14 in, 1 out]
          n521 = Unbundle By Name(w1421) -> ("code"=w1424:i32)
          n522 = case shown="No Error" w1421 {
            selector: w1421 -> [_ w1439]
            tunnel: [_ w1437] -> w1423
            frame No Error {
            }
            frame Error {
              n523 = Unbundle By Name(w1439) -> ("source"=w1438:string)
              n524 = call-poly "CoreLib.data 2 byte array.vi"("string"=w1438) -> ("byteArray out"=w1437:T1)  [unwired: 18 in]
            }
          }
          n525 = Bundle By Name(cluster=w1418, "Data"=w1423, "Error #"=w1424) -> (w1419:T2)
        }
        frame "_set_PSDB_Data" {
          n526 = call "CAEObj.unfold trend data.vi"("i ref in"=w1448, "raw trend data"=w1449) -> ("quality"=w1444:i32, "no link"=w1441:bool, "data"=w1443:i8[], "typeDescriptor"=w1440:string, "error out"=w1442:errorcluster)  [unwired: 9 in, 4 out]
          n527 = case shown="No Error" w1442 {
            tunnel: w1447 -> [w1468 w1508]
            tunnel: [w1467 w1507] -> w1446
            tunnel: [w1466 w1508] -> w1445
            tunnel: w1448 -> [w1464 w1507]
            tunnel: w1441 -> [w1459 _]
            tunnel: w1440 -> [w1460 _]
            tunnel: w1443 -> [w1461 _]
            tunnel: w1444 -> [w1458 _]
            frame No Error {
              n528 = call "PH_PSDBWriter.get Subsystem DIM Service.vi"("no link"=w1459, "typeDescriptor"=w1460, "data"=w1461, "quality"=w1458) -> ("PHELIX Subsystems"=w1457:T17)
              n529 = call "PH_PSDBWriter.check PSDB writing condition.vi"("i ref in"=w1464, "wanted Subsystem"=w1457, "error IO"=w1468) -> ("i ref out"=w1463:refnum<vi>, "write PSDB?"=w1462:bool, "error out"=w1465:errorcluster)  [unwired: 14 in]
              n530 = case shown="True" w1462 {
                tunnel: w1465 -> [w1469 w1479]
                tunnel: [w1470 w1471] -> w1467
                tunnel: [w1469 w1472] -> w1466
                tunnel: w1463 -> [w1470 w1481]
                frame False {
                }
                frame True {
                  n531 = call "PH_Sequencer.Shot over at Heads.vi"("i ref in"=w1481, "error in (no error)"=w1479) -> ("i ref out"=w1480:refnum<vi>, "Shot of all PUs passed"=w1477:bool, "error out"=w1478:errorcluster)  [unwired: 15 in]
                  n532 = case shown="False" w1477 {
                    tunnel: [w1486 w1503] -> w1476
                    tunnel: [w1484 w1501] -> w1475
                    tunnel: w1480 -> [w1489 w1500]
                    tunnel: w1478 -> [w1488 w1499]
                    frame False {
                      n533 = call "PH_Sequencer.get data to modify.vi"("i ref in"=w1489, "error in (no error)"=w1488) -> ("i ref out"=w1485:refnum<vi>, "i attribute"=w1482:T7, "timed out"=w1483:bool, "error out"=w1487:errorcluster)  [unwired: 14 in]
                      n534 = case shown="False" w1483 {
                        tunnel: w1487 -> [w1496 w1497]
                        tunnel: [w1495 w1497] -> w1486
                        tunnel: w1485 -> [w1494 w1498]
                        tunnel: [w1493 w1498] -> w1484
                        tunnel: w1482 -> [w1492 _]
                        frame False {
                          n535 = Bundle By Name(cluster=w1492, "PSDB.Write 2 early"=TRUE) -> (w1491:T7)
                          n536 = call "PH_Sequencer.set modified data.vi"("i ref in"=w1494, "i attribute"=w1491, "error in (no error)"=w1496) -> ("i ref out"=w1493:refnum<vi>, "error out"=w1495:errorcluster)  [unwired: 15 in]
                        }
                        frame True {
                        }
                      }
                    }
                    frame True {
                      n537 = call "PH_Sequencer.PC Write PSDB.vi"("i ref in"=w1500, "error IO"=w1499) -> ("i ref out"=w1506:refnum<vi>, "error out"=w1505:errorcluster)  [unwired: 16 in]
                      n538 = call "PH_PSDBWriter.evt call write PSDB.vi"("i ref in"=w1506, "error in (no error)"=w1505) -> ("i ref out"=w1502:refnum<vi>, "error out"=w1504:errorcluster)  [unwired: 16 in]
                      n539 = call "PH_Sequencer.set PSDB Data.vi"("i ref in"=w1502, "error in"=w1504) -> ("i ref out"=w1501:refnum<vi>, "error out"=w1503:errorcluster)  [unwired: 16 in]
                    }
                  }
                  n540 = call "PH_Sequencer.PC Write PSDB.vi"("i ref in"=w1475, "error IO"=w1476) -> ("i ref out"=w1474:refnum<vi>, "error out"=w1473:errorcluster)  [unwired: 16 in]
                  n541 = call "PH_PSDBWriter.evt call write PSDB.vi"("i ref in"=w1474, "error in (no error)"=w1473) -> ("i ref out"=w1471:refnum<vi>, "error out"=w1472:errorcluster)  [unwired: 16 in]
                }
              }
            }
            frame Error {
            }
          }
          n542 = call "BaseProcess.set event status.vi"("i ref in"=w1446, "EventStatus"=w1452, "error in (no error)"=w1445) -> ("i ref out"=w1454:refnum<vi>, "error out"=w1453:errorcluster)  [unwired: 14 in, 1 out]
          n543 = case shown="No Error" w1453 {
            selector: w1453 -> [_ w1511]
            tunnel: [_ w1509] -> w1455
            frame No Error {
            }
            frame Error {
              n544 = Unbundle By Name(w1511) -> ("source"=w1510:string)
              n545 = call-poly "CoreLib.data 2 byte array.vi"("string"=w1510) -> ("byteArray out"=w1509:T1)  [unwired: 18 in]
            }
          }
          n546 = Unbundle By Name(w1453) -> ("code"=w1456:i32)
          n547 = Bundle By Name(cluster=w1450, "Data"=w1455, "Error #"=w1456) -> (w1451:T2)
        }
        frame Default {
          w1516 = T18."PreAmp" ("Wanted State")
          w1518 = T18."MainAmp" ("Wanted State")
          # "In the default case, always call the ProcCase method of the parent class"
          n548 = call "PH_SystemInformation.get Enabling State.vi"("i ref in"=w1513, "Wanted State"=w1518, "error in (no error)"=w1512) -> ("i ref out"=w1520:refnum<vi>, "Enabling State"=w1517:T15, "error out"=w1522:errorcluster)  [unwired: 14 in]
          n549 = call "PH_SystemInformation.get Enabling State.vi"("i ref in"=w1520, "Wanted State"=w1516, "error in (no error)"=w1522) -> ("i ref out"=w1519:refnum<vi>, "Enabling State"=w1515:T15, "error out"=w1521:errorcluster)  [unwired: 14 in]
          n550 = call "PH_BeamlineController.ProcCases.vi"("i ref in"=w1519, "selector"=w1527, "Data"=w1514, "call cluster"=w1526, "error in (no error)"=w1521) -> ("i ref out"=w1528:refnum<vi>, "answer cluster"=w1524:T2, "error out"=w1525:errorcluster)  [unwired: 12 in]
          n551 = case shown="No Error" w1525 {
            selector: w1525 -> [w1548 _]
            tunnel: [w1532 w1569] -> w1530
            tunnel: [w1534 w1568] -> w1529
            tunnel: w1528 -> [w1547 w1567]
            tunnel: w1514 -> [_ w1566]
            tunnel: w1527 -> [_ w1565]
            tunnel: w1526 -> [_ w1564]
            tunnel: w1524 -> [w1549 _]
            tunnel: [w1549 w1562] -> w1523
            tunnel: w1521 -> [_ w1563]
            tunnel: w1518 -> [w1546 _]
            tunnel: w1517 -> [w1545 _]
            tunnel: w1516 -> [w1538 _]
            tunnel: w1515 -> [w1537 _]
            frame No Error {
              n552 = call "PH_SystemInformation.get Enabling State.vi"("i ref in"=w1547, "Wanted State"=w1546, "error in (no error)"=w1548) -> ("i ref out"=w1541:refnum<vi>, "Enabling State"=w1544:T15, "error out"=w1543:errorcluster)  [unwired: 14 in]
              n553 = Not Equal?(x=w1545, y=w1544) -> (x != y?=w1539:bool)
              n554 = case shown="False" w1539 {
                tunnel: w1543 -> [w1556 w1561]
                tunnel: [w1556 w1560] -> w1542
                tunnel: w1541 -> [w1557 w1559]
                tunnel: [w1557 w1558] -> w1540
                frame False {
                }
                frame True {
                  n555 = call "PH_Sequencer.PC SetPPMAGUIElements.vi"("i ref in"=w1559, "error in (no error)"=w1561) -> ("i ref out"=w1558:refnum<vi>, "error out"=w1560:errorcluster)  [unwired: 16 in]
                }
              }
              n556 = call "PH_SystemInformation.get Enabling State.vi"("i ref in"=w1540, "Wanted State"=w1538, "error in (no error)"=w1542) -> ("i ref out"=w1533:refnum<vi>, "Enabling State"=w1536:T15, "error out"=w1535:errorcluster)  [unwired: 14 in]
              n557 = Not Equal?(x=w1537, y=w1536) -> (x != y?=w1531:bool)
              n558 = case shown="False" w1531 {
                tunnel: w1535 -> [w1550 w1555]
                tunnel: [w1550 w1554] -> w1534
                tunnel: w1533 -> [w1551 w1553]
                tunnel: [w1551 w1552] -> w1532
                frame False {
                }
                frame True {
                  n559 = call "PH_Sequencer.PC SetPPPAGUIElements.vi"("i ref in"=w1553, "error in (no error)"=w1555) -> ("i ref out"=w1552:refnum<vi>, "error out"=w1554:errorcluster)  [unwired: 16 in]
                }
              }
            }
            frame Error {
              n560 = call "PH_PSDBWriter.ProcCases.vi"("i ref in"=w1567, "selector"=w1565, "Data"=w1566, "call cluster"=w1564, "error in"=w1563) -> ("i ref out"=w1569:refnum<vi>, "answer cluster"=w1562:T2, "error out"=w1568:errorcluster)  [unwired: 12 in]
            }
          }
        }
      }
    }
    frame Error {
    }
  }
  "answer cluster" <- w7
  "i ref out" <- w4
  "error out" <- w3
